vi "Main fref.vi"() -> ()   [LabVIEW 2014]
uses:
  <vilib>/Utility/config.llb/NI_LVConfig.lvlib
  <vilib>/Utility/config.llb/Write Key (String).vi
  <vilib>/Utility/miscctls.llb/LVBoundsTypeDef.ctl
  <vilib>/Utility/miscctls.llb/LVRowAndColumnTypeDef.ctl
  <vilib>/Utility/config.llb/Read Key (String).vi
  TcpConnect/Ctrl/Type.ctl
  user32.dll
  <vilib>/Instr/_visa.llb/VISA Configure Serial Port (Instr).vi
  <vilib>/vision/Image Controls.llb/IMAQ Image.ctl
panel:
  out "螺栓6读取错误":bool
  in  "螺栓6扭矩读取":bool
  in  "扫码保存图片过程":u8
  out "error out 9":errorcluster
  out "error out 8":errorcluster
  out "扭矩/角度":string[][](array[string])
  out "error out 7":errorcluster
  out "error out 5":errorcluster
  out "error out 6":errorcluster
  out "error out 3":errorcluster
  in  "启动python":dbl
  out "产品型号选择":i16
  out "螺栓数量":i16
  out "螺栓5读取错误":bool
  out "螺栓4读取错误":bool
  out "螺栓3读取错误":bool
  out "螺栓2读取错误":bool
  out "螺栓1读取错误":bool
  out "螺栓0读取错误":bool
  in  "螺栓0扭矩读取":bool
  in  "螺栓1扭矩读取":bool
  in  "螺栓2扭矩读取":bool
  in  "螺栓3扭矩读取":bool
  in  "螺栓4扭矩读取":bool
  in  "螺栓5扭矩读取":bool
  in  "复位":bool
  in  "拍照复位信号":bool
  in  "扫码复位信号":bool
  in  "扭矩保存过程":u8
  out "角度字符串":string
  out "扭矩字符串":string
  out "读到的数据":string
  in  "错误输入（无错误） 2":errorcluster caption="错误输入（无错误）"
  out "错误输出 2":errorcluster caption="错误输出"
  in  "拍照存储过程":u8
  in  "开始拍照":bool
  out "图片保存路径":string
  out "error out 4":errorcluster
  in  "Image":T1
  out "扫码NG":bool
  out "扫码OK":bool
  in  "扫码复位":bool
  in  "开始扫码":bool
  out "错误输出":errorcluster
  in  "错误输入（无错误）":errorcluster
  out "当日序号":string
  in  "记录流程":i8
  out "error out":errorcluster caption="错误输出"
  in  "活动单元格:活动单元格 5":T2 caption="活动单元格:活动单元格"
  in  "活动单元格:活动单元格 4":T2 caption="活动单元格:活动单元格"
  in  "活动单元格:活动单元格 3":T2 caption="活动单元格:活动单元格"
  in  "修改确认流程":dbl
  in  "登录过程":dbl
  in  "活动单元格:活动单元格":T2
  in  "选项卡控件":enum32{"操作页面", "设置页面"}(tab)
  out "扭矩7合格":bool
  out "正在拧紧图像（二维码绑定）":T1(plugin-control) caption="正在"
  in  "扭矩角度表格":string[][](table)
  out "拍照合格":bool
  out "扭矩5合格":bool
  out "扭矩6合格":bool
  out "今日合格":string
  out "今日总数":string
  in  "已选产品":string[][](table)
  in  "作业员 Operator":u16(ring) items=["张三", "", "", "", "", "", "", "", "", ""]
  out "二维码":string
  in  "表格":string[][](table)
  out "扭矩4合格":bool
  out "扭矩2合格":bool
  out "扭矩1合格":bool
  out "扭矩3合格":bool
  out "待拧紧前识别图像":T1(plugin-control)
  out "实时图像":T1(plugin-control)
  out "二维码长度":i32
  out "二维码对应程序号":i16
  in  "用户登录":bool
  in  "密码":string
  in  "用户名":string
  in  "用户退出":bool
  in  "产品参数列表（点击表格内任意位置，即可选中所对应产品）":string[][](table)
  in  "程序选择确定":bool
  in  "作业员列表":string[][](table)
  out "字符串":string
types:
  T1 = typedef "IMAQ Image.ctl" = refnum<image>
  T2 = typedef "LVRowAndColumnTypeDef.ctl" = cluster{"Row":i32, "Column":i32}
  T3 = typedef "Type.ctl" = enum16{"Init", "Loop", "Write", "Read", "Exit", "Open", "Close"}
  T4 = typedef "NI_LVConfig.lvlib/Config Data RefNum.ctl" = refnum<k1>
  T5 = cluster{"Name":string, "Type":enum16{"Line", "Broken Line", "Free Hand Line", "Rotated Rectangle", "Oval", "Polygon", "Free Hand", "Bitmap", "Text"}, "Coordinates":i32[], "Colors":u32[], "Drawing Mode":u32, "Text":string, "Results":cluster{"Process ID":string, "Measure":u16, "Name":string, "String Format":u16, "Width":i16, "Precision":i16, "True String":string, "False String":string}[], "Font, Size & Style":cluster{"Desired Font (Application)":enum16{"User-specified Font", "Application Font", "System Font", "Dialog Font"}, "[User-specified Font]":cluster{"Font Name":string, "Size":i16, "Strikeout?":bool, "Italic?":bool, "Underline?":bool, "Outline?":bool, "Shadow?":bool, "Bold?":bool, "Rotation Angle":dbl}, "Horizontal Alignment":i16, "Vertical Alignment":i16}, "Image File Path":path, "Use Keying Color":bool}[]
  T6 = cluster{"Global Rectangle":i32[], "Contours":cluster{"ID":enum32{"External", "Internal"}, "Type":u32, "Coordinates":i32[]}[]}
  T7 = cluster{"Name":string, "Type":enum16{"Line", "Broken Line", "Free Hand Line", "Rotated Rectangle", "Oval", "Polygon", "Free Hand", "Bitmap", "Text"}, "Coordinates":i32[], "Colors":u32[], "Drawing Mode":u32, "Text":string, "Results":cluster{"Process ID":string, "Measure":u16, "Name":string, "String Format":u16, "Width":i16, "Precision":i16, "True String":string, "False String":string}[], "Font, Size & Style":cluster{"Desired Font (Application)":enum16{"User-specified Font", "Application Font", "System Font", "Dialog Font"}, "[User-specified Font]":cluster{"Font Name":string, "Size":i16, "Strikeout?":bool, "Italic?":bool, "Underline?":bool, "Outline?":bool, "Shadow?":bool, "Bold?":bool, "Rotation Angle":dbl}, "Horizontal Alignment":i16, "Vertical Alignment":i16}, "Image File Path":path, "Use Keying Color":bool}
  T8 = enum16{"Line", "Broken Line", "Free Hand Line", "Rotated Rectangle", "Oval", "Polygon", "Free Hand", "Bitmap", "Text"}
  T9 = cluster{"Process ID":string, "Measure":u16, "Name":string, "String Format":u16, "Width":i16, "Precision":i16, "True String":string, "False String":string}[]
  T10 = cluster{"Desired Font (Application)":enum16{"User-specified Font", "Application Font", "System Font", "Dialog Font"}, "[User-specified Font]":cluster{"Font Name":string, "Size":i16, "Strikeout?":bool, "Italic?":bool, "Underline?":bool, "Outline?":bool, "Shadow?":bool, "Bold?":bool, "Rotation Angle":dbl}, "Horizontal Alignment":i16, "Vertical Alignment":i16}
  T11 = enum16{"Standard", "Buffered", "CRLF", "Immediate"}
  T12 = typedef "LVBoundsTypeDef.ctl" = cluster{"Width":u32, "Height":u32}
  T13 = typedef "LVPoint32TypeDef.ctl" = cluster{"Horizontal":i32, "Vertical":i32}
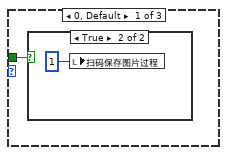
[diagram p2: hidden frame]
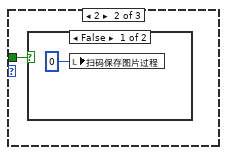
[diagram p4: hidden frame]
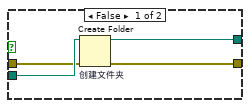
[diagram p6: hidden frame]
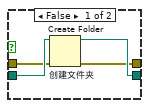
[diagram p7: hidden frame]
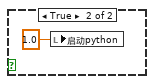
[diagram p8: hidden frame]
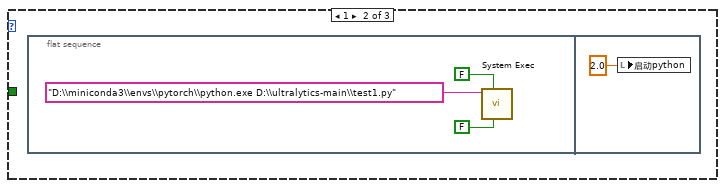
[diagram p9: hidden frame]
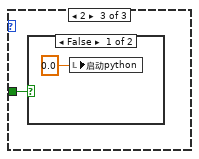
[diagram p10: hidden frame]
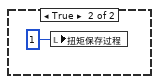
[diagram p14: hidden frame]
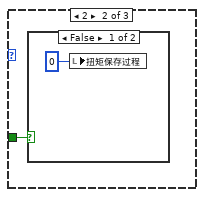
[diagram p15: hidden frame]
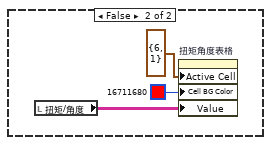
[diagram p18: hidden frame]
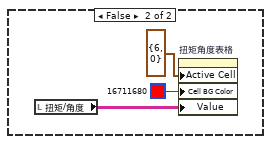
[diagram p19: hidden frame]
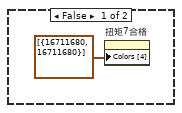
[diagram p20: hidden frame]
diagram:
  n1 = flat-sequence {
    frame #0 {
      w16 = 0
      w14 = 0 items=["NULL"]
      n2 = call "IMAQ Create"("Image Name"="untitled") -> ("New Image"=w25:T1, "error out"=w21:errorcluster)  [unwired: 4 in]
      n3 = call "IMAQ ReadFile 2"("File Path"=path "d:/aotecar.jpg", "error in (no error)"=w21, "Image"=w25) -> ("error out"=w22:errorcluster, "Image Out"=w24:T1)  [unwired: 4 in, 3 out]
      n4 = dll-call lib="user32.dll" fn="FindWindowA" label="FindWindow"("lpszClassName"=w14, "lpszWindowName"="Main.vi") -> ("hWnd"=w18:u32)  [unwired: 5 in, 2 out]
      n5 = call-poly "IMAQ Write File 2"("error in (no error)"=w22, "File Path"=path "d:/image.jpg", "Image"=w24) -> ("Image Out (duplicate)"=w19:T1)  [unwired: 7 in, 1 out]
      n6 = call <vilib>:"System Exec.vi"("run minimized? (F)"=TRUE, "wait until completion? (T)"=FALSE, "command line"="taskkill /F /IM python.exe") -> ()  [unwired: 5 in, 4 out]
      n7 = dll-call lib="USER32.DLL" fn="SetWindowPos"("hWnd"=w18, "hWndInsertAfter"=-1, "left"=w16, "top"=w16, "width"=w16, "height"=w16, "fuFlags"=u32 3) -> ()  [unwired: 11 in, 2 out]
      n8 = local write "待拧紧前识别图像"(w19) -> ()
    }
    frame #1 {
      n9 = Wait (ms)(milliseconds to wait=u32 2000 ("等待时间（毫秒）")) -> ()  [unwired: 1 out]
    }
    frame #2 {
      n10 = while {
        stop <- FALSE stop-if-true
        n11 = call "Get Task List 2.vi"() -> ("names of application windows"=w37:string[])  [unwired: 6 in, 1 out]
        n12 = for {
          N: 10 -> [_]
          tunnel: w37 -> [w47]
          shift-right: [w41] -> w35
          shift-left: 0 -> [w42]
          i -> [w40]
          n13 = Index Array(array=w47, index=w40) -> (element=w46:string)
          n14 = Search and Replace String(case sensitive?=TRUE ("忽略大小写？(F)"), input string=w46, search string="python" ("搜索字符串")) -> (number of replacements=w43:i32)  [unwired: 5 in, 3 out]
          n15 = Add(x=w42, y=w43) -> (x+y=w41:i32)
        }
        n16 = Wait (ms)(milliseconds to wait=u32 1000 ("等待时间（毫秒）")) -> ()  [unwired: 1 out]
        n17 = Equal?(x=w35, y=0) -> (x = y?=w33:bool)
        n18 = case shown="0, 默认" "启动python" {
          tunnel: w33 -> [w48 _ w54]
          frame 0, Default {
            n19 = case shown="False" w48 {
              frame False {
              }
              frame True {
                n20 = local write "启动python"(1.0 ("启动python")) -> ()
              }
            }
          }
          frame 1 {
            n21 = flat-sequence {
              frame #0 {
                n22 = call <vilib>:"System Exec.vi"("run minimized? (F)"=FALSE, "wait until completion? (T)"=FALSE, "command line"="D:\\miniconda3\\envs\\pytorch\\python.exe D:\\ultralytics-main\\test1.py") -> ()  [unwired: 5 in, 4 out]
              }
              frame #1 {
                n23 = local write "启动python"(2.0 ("启动python")) -> ()
              }
            }
          }
          frame 2 {
            n24 = case shown="False" w54 {
              frame False {
                n25 = local write "启动python"(0.0 ("启动python")) -> ()
              }
              frame True {
              }
            }
          }
        }
      }
    }
  }
  n26 = while {
    stop <- FALSE stop-if-true
    n27 = Wait (ms)(milliseconds to wait=u32 100 ("等待时间（毫秒）")) -> ()  [unwired: 1 out]
    n28 = case shown="0, 默认" "修改确认流程" {
      tunnel: "程序选择确定" -> [w60 _ w136]
      frame 0, Default {
        n29 = case shown="False" w60 {
          frame False {
          }
          frame True {
            n30 = local write "修改确认流程"(1.0 ("修改确认流程")) -> ()
          }
        }
      }
      frame 1 {
        n31 = flat-sequence {
          tunnel: [w70] -> w67
          tunnel: [w69] -> w66
          tunnel: w67 -> [w100]
          tunnel: w66 -> [w99]
          tunnel: [w98] -> w65
          tunnel: [w97] -> w64
          tunnel: w65 -> [w132]
          tunnel: w64 -> [w131]
          tunnel: [w131] -> w63
          tunnel: [w132] -> w62
          tunnel: w63 -> [w134]
          tunnel: w62 -> [w133]
          frame #0 {
            n32 = property on="产品参数列表（点击表格内任意位置，即可选中所对应产品）" class="Tbl (严格)"() -> ("Column Headers[]"=w71:string[])  [unwired: 2 in, 2 out]
            n33 = Array Size(array=w71) -> (size(s)=w72:i32)
            n34 = call <vilib>:"Open Config Data.vi"("create file if necessary (T)"=TRUE, "configuration file path"=path "D:/Setup.ini") -> ("error out"=w73:errorcluster, "refnum"=w75:T4)  [unwired: 7 in, 1 out]
            n35 = for {
              N: w72 -> [_]
              tunnel: w75 -> [w82]
              tunnel: w73 -> [w81]
              tunnel: w71 -> [w80]
              tunnel: [w78] -> w70
              tunnel: [w77] -> w69
              i -> [w76]
              n36 = Index Array(array=w80, index=w76) -> (element=w79:string)
              n37 = for {
                N: 100 -> [_]
                tunnel: w82 -> [w96]
                tunnel: [w94] -> w78
                tunnel: w81 -> [w93]
                tunnel: [w92] -> w77
                tunnel: w79 -> [w86]
                tunnel: w76 -> [w85]
                i -> [w91]
                n38 = local read "产品参数列表（点击表格内任意位置，即可选中所对应产品）"() -> (w84:string[][])
                n39 = Increment(x=w91) -> (x+1=w90:i32)
                n40 = Number To Decimal String(number=w90) -> (decimal integer string=w89:string)  [unwired: 1 in]
                n41 = Concatenate Strings(w86, w89) -> (w88:string)
                n42 = Index Array(array=w84, index (row)=w91, index (col)=w85) -> (element=w87:string)
                n43 = call-poly <vilib>:"Write Key.vi"("section"="Setup", "error in (no error)"=w93, "value"=w87, "key"=w88, "refnum"=w96) -> ("error out"=w92:errorcluster, "refnum out"=w94:T4)  [unwired: 4 in, 1 out]
              }
            }
          }
          frame #1 {
            n44 = for {
              N: 35 -> [_]
              tunnel: w100 -> [w130]
              tunnel: [w127] -> w103
              tunnel: w99 -> [w126]
              tunnel: [w125] -> w104
              i -> [w124]
              n45 = Increment(x=w124) -> (x+1=w122:i32)
              n46 = Number To Decimal String(number=w122) -> (decimal integer string=w121:string)  [unwired: 1 in]
              n47 = Concatenate Strings("作业员编码" ("字符串"), w121) -> (w120:string)
              n48 = Index Array(array="作业员列表", index (row)=w124, index (col)=0 ("Column")) -> (element=w118:string)
              n49 = call-poly <vilib>:"Write Key.vi"("section"="Setup", "error in (no error)"=w126, "value"=w118, "key"=w120, "refnum"=w130) -> ("error out"=w125:errorcluster, "refnum out"=w127:T4)  [unwired: 4 in, 1 out]
            }
            n50 = for {
              N: 35 -> [_]
              tunnel: w103 -> [w117]
              tunnel: [w114] -> w98
              tunnel: w104 -> [w113]
              tunnel: [w112] -> w97
              i -> [w111]
              n51 = Increment(x=w111) -> (x+1=w109:i32)
              n52 = local read "作业员列表"() -> (w106:string[][])
              n53 = Number To Decimal String(number=w109) -> (decimal integer string=w108:string)  [unwired: 1 in]
              n54 = Concatenate Strings("作业员姓名" ("字符串"), w108) -> (w107:string)
              n55 = Index Array(array=w106, index (row)=w111, index (col)=1 ("Column")) -> (element=w105:string)
              n56 = call-poly <vilib>:"Write Key.vi"("section"="Setup", "error in (no error)"=w113, "value"=w105, "key"=w107, "refnum"=w117) -> ("error out"=w112:errorcluster, "refnum out"=w114:T4)  [unwired: 4 in, 1 out]
            }
          }
          frame #2 {
          }
          frame #3 {
            n57 = call <vilib>:"Close Config Data.vi"("error in (no error)"=w134, "refnum"=w133) -> ()  [unwired: 8 in, 2 out]
          }
          frame #4 {
            n58 = local write "修改确认流程"(2.0 ("修改确认流程")) -> ()
          }
        }
      }
      frame 2 {
        n59 = case shown="False" w136 {
          frame False {
            n60 = local write "修改确认流程"(0.0 ("修改确认流程")) -> ()
          }
          frame True {
          }
        }
      }
    }
  }
  n61 = disable-structure shown="已启用" {
    frame Disabled {
      n62 = flat-sequence {
        tunnel: [w143] -> w139
        tunnel: [w142] -> w138
        tunnel: w139 -> [w152]
        tunnel: w138 -> [w151]
        frame #0 {
          n63 = call <vilib>:"Open Config Data.vi"("create file if necessary (T)"=TRUE, "configuration file path"=path "D:/Test/Setup.ini") -> ("error out"=w149:errorcluster, "refnum"=w148:T4)  [unwired: 7 in, 1 out]
          n64 = call-poly <vilib>:"Read Key.vi"("section"="Setup", "error in (no error)"=w149, "refnum"=w148) -> ("error out"=w143:errorcluster, "value"=w147:string, "refnum out"=w142:T4, "key"=w140:string)  [unwired: 4 in, 1 out]
          n65 = Write to Text File(file (use dialog)=path "D:/扫码端口号.txt" ("文件（使用对话框）"), text=w147) -> ()  [unwired: 2 in, 3 out]
        }
        frame #1 {
          n66 = call <vilib>:"Close Config Data.vi"("error in (no error)"=w152, "refnum"=w151) -> ("error out"=→"error out":errorcluster)  [unwired: 8 in, 1 out]
        }
        frame #2 {
          n67 = Wait (ms)(milliseconds to wait=u32 2000 ("等待时间（毫秒）")) -> ()  [unwired: 1 out]
        }
        frame #3 {
          n68 = while {
            stop <- w158 stop-if-true
            n69 = Read from Text File(file (use dialog)=path "D:/扫码端口号.txt" ("文件（使用对话框）")) -> (text=w154:string)  [unwired: 3 in, 3 out]
            n70 = VISA Open(VISA resource name=w154) -> (VISA resource name=w156:refnum<visa-resource-name>, error out=w157:errorcluster)  [unwired: 4 in]
            n71 = case shown="错误" w157 {
              tunnel: w156 -> [w187 _]
              tunnel: 9600 -> [w183 _]
              tunnel: [w182 _] -> w162
              tunnel: [w181 _] -> w161
              frame No Error {
                n72 = call-poly "VISA Configure Serial Port"("VISA resource name"=w187, "baud rate (9600)"=w183) -> ("VISA resource name out"=w185:refnum<visa-resource-name>, "error out"=w186:errorcluster)  [unwired: 12 in]
                n73 = VISA Set I/O Buffer Size "VISA设置I/O缓冲区大小"(VISA resource name=w185, size (4096)=u32 20480 ("大小(4096)"), error in (no error)=w186) -> (VISA resource name out=w182:refnum<visa-resource-name>, error out=w181:errorcluster)  [unwired: 1 in]
              }
              frame Error {
                n74 = One Button Dialog(message="ERROR！" ("消息")) -> ()  [unwired: 1 in, 1 out]
              }
            }
            n75 = while {
              tunnel: w162 -> [w166]
              tunnel: w161 -> [w165]
              tunnel: [w172] -> w160
              tunnel: [w171] -> w159
              shift-right: [w170] -> _
              shift-left: _ -> [w169]
              tunnel: [w167] -> w158
              stop <- w167 stop-if-true
              w167 = FALSE
              n76 = Concatenate Strings "连接字符串"(w169) -> (w164:string)  [unwired: 1 in]
              n77 = flat-sequence {
                tunnel: w166 -> [w180]
                tunnel: w165 -> [w179]
                tunnel: [w175] -> w172
                tunnel: [w174] -> w171
                tunnel: [w173] -> w170
                frame #0 {
                  n78 = property class="Instr"(reference=w180, error in=w179) -> (reference out=w178:refnum<visa-resource-name>, error out=w177:errorcluster, "Bytes at Port"=w176:u32)
                  n79 = VISA Read(VISA resource name=w178, byte count=w176, error in (no error)=w177) -> (VISA resource name out=w175:refnum<visa-resource-name>, read buffer=w173:string, error out=w174:errorcluster)  [unwired: 1 out]
                }
              }
              n80 = local write item#-1(w164) -> ()
              n81 = Wait Until Next ms Multiple(millisecond multiple=u32 2 ("毫秒倍数")) -> ()  [unwired: 1 out]
            }
            n82 = VISA Close(VISA resource name=w160, error in (no error)=w159) -> ()  [unwired: 1 out]
          }
        }
      }
    }
    frame Enabled {
    }
  }
  n83 = disable-structure shown="禁用" {
    frame Disabled {
      n84 = while {
        stop <- FALSE stop-if-true
        n85 = local read item#-1() -> (w189)
        n86 = case shown="1" "记录流程" {
          tunnel: w189 -> [w192 _ w288]
          frame 0 {
            n87 = case shown="False" w192 {
              frame False {
              }
              frame True {
                n88 = local write "记录流程"(i8 1 ("耐压测试左")) -> ()
              }
            }
          }
          frame 1 {
            n89 = flat-sequence {
              tunnel: [w198] -> w195
              tunnel: w195 -> [w208]
              tunnel: [w238] -> w194
              tunnel: w194 -> [w273]
              frame #0 {
                n90 = Open/Create/Replace File(file path (use dialog)=path "D:/日期.txt" ("文件（使用对话框）")) -> (refnum out=w205:refnum<file>, error out=w204:errorcluster)  [unwired: 5 in, 1 out]
                n91 = Read from Text File "读取文本文件"(file (use dialog)=w205, error in=w204) -> (refnum out=w197:refnum<file>, text=w201:string, error out=w196:errorcluster)  [unwired: 2 in, 1 out]
                n92 = Close File(refnum=w197, error in=w196) -> ()  [unwired: 2 out]
                n93 = Format Date/Time String(time format string (%c)="%Y%m%d" ("时间格式字符串(%c)")) -> (date/time string=w202:string)  [unwired: 2 in]
                n94 = Decimal String To Number(string=w201) -> (number=w199:i32)  [unwired: 2 in, 1 out]
                n95 = Decimal String To Number(string=w202) -> (number=w200:i32)  [unwired: 2 in, 1 out]
                n96 = Equal?(x=w199, y=w200) -> (x = y?=w198:bool)
              }
              frame #1 {
                n97 = case shown="True" w208 {
                  tunnel: [w209 w221] -> w207
                  frame False {
                    n98 = Number To Decimal String(number=1 ("数字"), width (-)=i16 4 ("宽度(-)")) -> (decimal integer string=w219:string)
                    n99 = call <vilib>:"Space Constant.vi"() -> ("String"=w220:string)
                    n100 = Search and Replace String(replace all?=TRUE ("替换全部？(F)"), input string=w219, search string=w220, replace string="0" ("替换字符串(\"\")")) -> (result string=w209:string)  [unwired: 4 in, 3 out]
                    n101 = Open/Create/Replace File(file path (use dialog)=path "D:/序号.txt" ("文件（使用对话框）")) -> (refnum out=w212:refnum<file>, error out=w211:errorcluster)  [unwired: 5 in, 1 out]
                    n102 = Write to Text File "写入文本文件"(file (use dialog)=w212, text=w209, error in=w211) -> (refnum out=w217:refnum<file>, error out=w218:errorcluster)  [unwired: 1 in, 1 out]
                    n103 = Close File(refnum=w217, error in=w218) -> ()  [unwired: 2 out]
                  }
                  frame True {
                    n104 = Open/Create/Replace File(file path (use dialog)=path "D:/序号.txt" ("文件（使用对话框）")) -> (refnum out=w224:refnum<file>, error out=w225:errorcluster)  [unwired: 5 in, 1 out]
                    n105 = Read from Text File "读取文本文件"(file (use dialog)=w224, error in=w225) -> (refnum out=w222:refnum<file>, text=w229:string, error out=w223:errorcluster)  [unwired: 2 in, 1 out]
                    n106 = Decimal String To Number(string=w229) -> (number=w235:i32)  [unwired: 2 in, 1 out]
                    n107 = Increment(x=w235) -> (x+1=w236:i32)
                    n108 = Number To Decimal String(number=w236, width (-)=i16 4 ("宽度(-)")) -> (decimal integer string=w231:string)
                    n109 = call <vilib>:"Space Constant.vi"() -> ("String"=w234:string)
                    n110 = Search and Replace String(replace all?=TRUE ("替换全部？(F)"), input string=w231, search string=w234, replace string="0" ("替换字符串(\"\")")) -> (result string=w221:string)  [unwired: 4 in, 3 out]
                    n111 = Write to Text File "写入文本文件"(file (use dialog)=w222, text=w221, error in=w223) -> (refnum out=w227:refnum<file>, error out=w228:errorcluster)  [unwired: 1 in, 1 out]
                    n112 = Close File(refnum=w227, error in=w228) -> ()  [unwired: 2 out]
                  }
                }
                "当日序号" <- w207
              }
              frame #2 {
                n113 = Build Path "创建路径"(name or relative path=path "D:/Image" ("基路径")) -> (appended path=w239:path)  [unwired: 1 in]
                n114 = call <vilib>:"Check if File or Folder Exists.vi"("path"=w239) -> ("error out"=w242:errorcluster, "file or folder exists?"=w241:bool, "dup path"=w240:path)  [unwired: 1 in, 7 out]
                n115 = case shown="True" w241 {
                  tunnel: [w243 w246] -> w238
                  tunnel: w240 -> [w245 w246]
                  tunnel: w242 -> [w244 _]
                  frame False {
                    n116 = Create Folder "创建文件夹"(path (use dialog)=w245, error in=w244) -> (created path=w243:path)  [unwired: 3 out]
                  }
                  frame True {
                  }
                }
              }
              frame #3 {
                n117 = Get Date/Time In Seconds "获取日期/时间（秒）"() -> (seconds since 1Jan1904=w271:timestamp)
                n118 = Format Date/Time String(time format string (%c)="%Y%m%d" ("时间格式字符串(%c)")) -> (date/time string=w248:string)  [unwired: 2 in]
                n119 = Open/Create/Replace File(file path (use dialog)=path "D:/日期.txt" ("文件（使用对话框）")) -> (refnum out=w250:refnum<file>, error out=w251:errorcluster)  [unwired: 5 in, 1 out]
                n120 = Path To String(path=w273) -> (string=w281:string)
                n121 = Write to Text File(file (use dialog)=w250, text=w248, error in=w251) -> (refnum out=w253:refnum<file>, error out=w254:errorcluster)  [unwired: 1 in, 1 out]
                n122 = Format Date/Time String(time format string (%c)="%Y-%m-%d" ("时间格式字符串(%c)"), seconds (now)=w271) -> (date/time string=w276:string)  [unwired: 1 in]
                n123 = Close File(refnum=w253, error in=w254) -> ()  [unwired: 2 out]
                n124 = Concatenate Strings(w281, "\\", w276) -> (w275:string)
                n125 = Build Path(name or relative path=w275) -> (appended path=w277:path)  [unwired: 1 in]
                n126 = call <vilib>:"Check if File or Folder Exists.vi"("path"=w277) -> ("error out"=w280:errorcluster, "file or folder exists?"=w279:bool, "dup path"=w278:path)  [unwired: 1 in, 7 out]
                n127 = case shown="False" w279 {
                  tunnel: [w282 w285] -> w264
                  tunnel: w278 -> [w284 w285]
                  tunnel: w280 -> [w283 _]
                  frame False {
                    n128 = Create Folder(path (use dialog)=w284, error in=w283) -> (created path=w282:path)  [unwired: 3 out]
                  }
                  frame True {
                  }
                }
                n129 = Path To String(path=w264) -> (string=w256:string)
                n130 = Format Date/Time String(time format string (%c)="%Y-%m-%d-%H-%M-%S-翅片" ("时间格式字符串(%c)")) -> (date/time string=w262:string)  [unwired: 2 in]
                n131 = Format Date/Time String(time format string (%c)="%Y-%m-%d-%H-%M-%S-O型圈" ("时间格式字符串(%c)")) -> (date/time string=w259:string)  [unwired: 2 in]
                n132 = Concatenate Strings(w256, "\\", w262) -> (w265:string)
                n133 = Concatenate Strings(w256, "\\", w259) -> (w260:string)
                n134 = Build Path(name or relative path=w265) -> (appended path=w261:path)  [unwired: 1 in]
                n135 = Build Path(name or relative path=w260) -> (appended path=w255:path)  [unwired: 1 in]
                n136 = call-poly "IMAQ Write File 2"("File Path"=w261, "Image"="Image") -> ("error out"=w269:errorcluster, "Image Out (duplicate)"=w270:T1)  [unwired: 8 in]
                n137 = call-poly "IMAQ Write File 2"("File Path"=w255, "Image"="Image") -> ("error out"=w268:errorcluster, "Image Out (duplicate)"=w267:T1)  [unwired: 8 in]
                n138 = call "IMAQ Dispose"("Image"=w270, "error in (no error)"=w269) -> ()  [unwired: 4 in, 1 out]
                n139 = call "IMAQ Dispose"("Image"=w267, "error in (no error)"=w268) -> ()  [unwired: 4 in, 1 out]
              }
              frame #4 {
                n140 = Wait (ms)(milliseconds to wait=u32 1000 ("等待时间（毫秒）")) -> ()  [unwired: 1 out]
              }
              frame #5 {
              }
              frame #6 {
                n141 = local write "记录流程"(i8 2 ("耐压测试左")) -> ()
              }
            }
          }
          frame 2, Default {
            n142 = case shown="True" w288 {
              frame False {
                n143 = local write "记录流程"(i8 0 ("耐压测试左")) -> ()
              }
              frame True {
              }
            }
          }
        }
      }
    }
    frame Enabled {
    }
  }
  n144 = while {
    tunnel: [w296] -> w5
    tunnel: [w295] -> w4
    stop <- w299 stop-if-true
    w303 = u32 0 items=["Grayscale", "Binary", "Gradient", "Rainbow", "Temperature", "User Defined", "Binary 16 Bit", "Gradient 16 Bit", "Rainbow 16 Bit", "Temperature 16 Bit", "User Defined 16 Bit"] ("Palette Type")
    w304 = T6 {"Global Rectangle"=[545, -12, 2261, 2048], "Contours"=[{"ID"=enum."External", "Type"=3, "Coordinates"=[545, -12, 2261, 2048]}]}  # ROI Descriptor
    n145 = Wait (ms)(milliseconds to wait=u32 150 ("等待时间（毫秒）")) -> ()  [unwired: 1 out]
    n146 = Index Array(array=T5 [{"Name"="Text 1", "Type"=enum."Text", "Coordinates"=[900, 1900], "Colors"=[16711680, 16777216], "Drawing Mode"=0, "Text"="%Y%m%d_%H_%M_%Sour Text", "Results"=[], "Font, Size & Style"={"Desired Font (Application)"=enum."User-specified Font", "[User-specified Font]"={"Font Name"="Tahoma", "Size"=100, "Strikeout?"=FALSE, "Italic?"=FALSE, "Underline?"=FALSE, "Outline?"=FALSE, "Shadow?"=FALSE, "Bold?"=FALSE, "Rotation Angle"=0.0}, "Horizontal Alignment"=0, "Vertical Alignment"=0}, "Image File Path"=path "", "Use Keying Color"=FALSE}] ("Parameters"), index=0 ("索引")) -> (element=w311:T7)
    n147 = Unbundle By Name(w311) -> ("Name"=w312:string, "Type"=w313:T8, "Coordinates"=w314:i32[], "Colors"=w315:u32[], "Drawing Mode"=w316:u32, "Results"=w319:T9, "Font, Size & Style"=w320:T10, "Image File Path"=w321:path, "Use Keying Color"=w322:bool)  [unwired: 1 out]
    n148 = Format Date/Time String(time format string (%c)="%Y%m%d_%H_%M_%S" ("时间格式字符串(%c)")) -> (date/time string=w317:string)  [unwired: 2 in]
    n149 = Bundle By Name(cluster=w311, "Name"=w312, "Type"=w313, "Coordinates"=w314, "Colors"=w315, "Drawing Mode"=w316, "Text"=w317, "Results"=w319, "Font, Size & Style"=w320, "Image File Path"=w321, "Use Keying Color"=w322) -> (w323:T7)
    n150 = call "Vision Acquisition"() -> ("Image Out"=w301:T1, "Stopped"=w299:bool, "error out"=w300:errorcluster)  [unwired: 25 in]
    n151 = Build Array(w323) -> (w324:T5)
    n152 = call <vilib>:"IVA Mask from ROI.vi"("Shrink"=TRUE, "ROI Descriptor"=w304, "error in (no error)"=w300, "Out / In"=FALSE, "Image Src"=w301) -> ("error out"=w308:errorcluster, "Image Out"=w307:T1)  [unwired: 5 out]
    n153 = call <vilib>:"IVA Overlay - Overlay.vi"("error in (no error)"=w308, "Parameters"=w324, "Image In"=w307) -> ("error out"=w291:errorcluster, "Image Out"=w293:T1)  [unwired: 7 out]
    n154 = call "IMAQ Merge Overlay"("error in (no error)"=w291, "Image Src"=w293) -> ("error out"=w290:errorcluster, "Image Dst Out"=w292:T1)  [unwired: 8 in]
    "实时图像" <- w292
    n155 = property on="实时图像" class="ImageControl"(error in=w290, "Palette:Palette Type"=w303) -> (error out=→"error out 7":errorcluster)  [unwired: 1 in, 1 out]
    n156 = call-poly "IMAQ Write File 2"("Image Quality"=u32 250, "File Path"=path "d:/source.jpg", "Image"=w292) -> ("error out"=w296:errorcluster, "Image Out (duplicate)"=w295:T1)  [unwired: 7 in]
  }
  n157 = while {
    tunnel: [w326] -> w2
    tunnel: [w325] -> w1
    stop <- FALSE stop-if-true
    n158 = Wait (ms)(milliseconds to wait=u32 100 ("等待时间（毫秒）")) -> ()  [unwired: 1 out]
    n159 = local read "扫码OK"() -> (w327:bool)
    n160 = case shown="1" "扫码保存图片过程" {
      tunnel: w327 -> [w331 w333 _]
      tunnel: [_ _ w336] -> w326
      tunnel: [_ _ w335] -> w325
      frame 0, Default {
        n161 = case shown="True" w331 {
          frame False {
          }
          frame True {
            n162 = local write "扫码保存图片过程"(u8 1 ("扫码保存图片过程")) -> ()
          }
        }
      }
      frame 2 {
        n163 = case shown="False" w333 {
          frame False {
            n164 = local write "扫码保存图片过程"(u8 0 ("扫码保存图片过程")) -> ()
          }
          frame True {
          }
        }
      }
      frame 1 {
        n165 = flat-sequence {
          tunnel: [w361] -> w336
          tunnel: [w360] -> w335
          frame #0 {
            w338 = FALSE
            n166 = Initialize Array("", 7 ("维数大小"), 2 ("维数大小")) -> (w349:string[][])
            n167 = for {
              N: 7 -> [_]
              i -> [w350]
              n168 = for {
                N: 2 -> [_]
                tunnel: w350 -> [w357]
                i -> [w358]
                n169 = Bundle(w357, w358) -> (w356:cluster{i32, i32})  [unwired: 1 in]
                n170 = Initialize Array("", 7 ("维数大小"), 2 ("维数大小")) -> (w354:string[][])
                n171 = property on="扭矩角度表格" class="Tbl (严格)"("Active Cell"=w356, "Cell BG Color"=u32 16448250 ("活动单元格:单元格背景色"), "Value"=w354) -> ()  [unwired: 2 in, 2 out]
              }
            }
            n172 = local write "扭矩1合格"(w338) -> ()
            n173 = local write "扭矩2合格"(w338) -> ()
            n174 = local write "扭矩3合格"(w338) -> ()
            n175 = local write "扭矩4合格"(w338) -> ()
            n176 = local write "扭矩5合格"(w338) -> ()
            n177 = local write "扭矩6合格"(w338) -> ()
            n178 = property on="扭矩6合格" class="Bool (严格)"("Colors [4]"=cluster{u32, u32}[] [{12369084, 12369084}] ("颜色[4]")) -> ()  [unwired: 2 in, 2 out]
            n179 = local write "扭矩/角度"(w349) -> ()
            n180 = property on="扭矩4合格" class="Bool (严格)"("Colors [4]"=cluster{u32, u32}[] [{12369084, 12369084}] ("颜色[4]")) -> ()  [unwired: 2 in, 2 out]
            n181 = property on="扭矩5合格" class="Bool (严格)"("Colors [4]"=cluster{u32, u32}[] [{12369084, 12369084}] ("颜色[4]")) -> ()  [unwired: 2 in, 2 out]
            n182 = property on="扭矩3合格" class="Bool (严格)"("Colors [4]"=cluster{u32, u32}[] [{12369084, 12369084}] ("颜色[4]")) -> ()  [unwired: 2 in, 2 out]
            n183 = property on="扭矩2合格" class="Bool (严格)"("Colors [4]"=cluster{u32, u32}[] [{12369084, 12369084}] ("颜色[4]")) -> ()  [unwired: 2 in, 2 out]
            n184 = property on="扭矩1合格" class="Bool (严格)"("Colors [4]"=cluster{u32, u32}[] [{12369084, 12369084}] ("颜色[4]")) -> ()  [unwired: 2 in, 2 out]
            n185 = local write "扭矩7合格"(w338) -> ()
            n186 = property on="扭矩7合格" class="Bool (严格)"("Colors [4]"=cluster{u32, u32}[] [{12369084, 12369084}] ("颜色[4]")) -> ()  [unwired: 2 in, 2 out]
          }
          frame #1 {
            n187 = String To Path(string="D:\\Image\\" ("字符串")) -> (path=w400:path)
            n188 = Format Date/Time String(time format string (%c)="%Y%m") -> (date/time string=w399:string)  [unwired: 2 in]
            n189 = Build Path(base path=w400, name or relative path=w399) -> (appended path=w398:path)
            n190 = call <vilib>:"Check if File or Folder Exists.vi"("path"=w398) -> ("error out"=w405:errorcluster, "file or folder exists?"=w397:bool)  [unwired: 8 in, 1 out]
            n191 = case shown="True" w397 {
              tunnel: w398 -> [w420 w422]
              tunnel: [w419 w422] -> w403
              tunnel: w405 -> [w418 w421]
              tunnel: [w417 w421] -> w406
              frame False {
                n192 = Create Folder "创建文件夹"(path (use dialog)=w420, error in=w418) -> (created path=w419:path, error out=w417:errorcluster)  [unwired: 1 in, 1 out]
              }
              frame True {
              }
            }
            n193 = Format Date/Time String(time format string (%c)="%d") -> (date/time string=w402:string)  [unwired: 2 in]
            n194 = Build Path(base path=w403, name or relative path=w402) -> (appended path=w404:path)
            n195 = Index Array(array=T5 [{"Name"="Text 1", "Type"=enum."Text", "Coordinates"=[100, 2000], "Colors"=[16711680, 16777216], "Drawing Mode"=0, "Text"="%Y%m%d_%H_%M_%Sour Text", "Results"=[], "Font, Size & Style"={"Desired Font (Application)"=enum."User-specified Font", "[User-specified Font]"={"Font Name"="Tahoma", "Size"=100, "Strikeout?"=FALSE, "Italic?"=FALSE, "Underline?"=FALSE, "Outline?"=FALSE, "Shadow?"=FALSE, "Bold?"=FALSE, "Rotation Angle"=0.0}, "Horizontal Alignment"=0, "Vertical Alignment"=0}, "Image File Path"=path "", "Use Keying Color"=FALSE}] ("Parameters"), index=0 ("索引")) -> (element=w374:T7)
            n196 = Unbundle By Name(w374) -> ("Name"=w375:string, "Type"=w376:T8, "Coordinates"=w377:i32[], "Colors"=w378:u32[], "Drawing Mode"=w379:u32, "Results"=w380:T9, "Font, Size & Style"=w381:T10, "Image File Path"=w382:path, "Use Keying Color"=w383:bool)  [unwired: 1 out]
            n197 = call <vilib>:"Check if File or Folder Exists.vi"("error in (no error)"=w406, "path"=w404) -> ("error out"=w407:errorcluster, "file or folder exists?"=w401:bool)  [unwired: 7 in, 1 out]
            n198 = local read "二维码长度"() -> (w364:i32)
            n199 = case shown="True" w401 {
              tunnel: w404 -> [w414 w415]
              tunnel: [w413 w415] -> w395
              tunnel: w407 -> [w412 w416]
              tunnel: [w411 w416] -> _
              frame False {
                n200 = Create Folder "创建文件夹"(path (use dialog)=w414, error in=w412) -> (created path=w413:path, error out=w411:errorcluster)  [unwired: 1 in, 1 out]
              }
              frame True {
              }
            }
            n201 = local read "二维码"() -> (w365:string)
            n202 = local read "二维码"() -> (w369:string)
            n203 = Bundle By Name(cluster=w374, "Name"=w375, "Type"=w376, "Coordinates"=w377, "Colors"=w378, "Drawing Mode"=w379, "Text"=w369, "Results"=w380, "Font, Size & Style"=w381, "Image File Path"=w382, "Use Keying Color"=w383) -> (w384:T7)
            n204 = String Subset(string=w365, length (rest)=w364) -> (substring=w366:string)  [unwired: 1 in]
            n205 = Format Date/Time String(time format string (%c)="%Y%m%d_%H_%M_%S") -> (date/time string=w394:string)  [unwired: 2 in]
            n206 = call "IMAQ Create"("Image Name"="untitled3") -> ("New Image"=w409:T1, "error out"=w410:errorcluster)  [unwired: 4 in]
            n207 = Build Array(w384) -> (w385:T5)
            n208 = call "IMAQ ReadFile 2"("File Path"=path "d:/buffer.jpg", "error in (no error)"=w410, "Image"=w409) -> ("error out"=w362:errorcluster, "Image Out"=w363:T1)  [unwired: 4 in, 3 out]
            n209 = call <vilib>:"IVA Overlay - Overlay.vi"("error in (no error)"=w362, "Parameters"=w385, "Image In"=w363) -> ("error out"=w372:errorcluster, "Image Out"=w373:T1)  [unwired: 7 out]
            n210 = Concatenate Strings(w366, w394, ".JPEG" ("字符串")) -> (w408:string)
            n211 = Build Path(base path=w395, name or relative path=w408) -> (appended path=w393:path)
            n212 = call "IMAQ Merge Overlay"("error in (no error)"=w372, "Image Src"=w373) -> ("error out"=w367:errorcluster, "Image Dst Out"=w368:T1)  [unwired: 8 in]
            n213 = Path To String(path=w393) -> (string=→"图片保存路径":string)
            n214 = call-poly "IMAQ Write File 2"("error in (no error)"=w367, "File Path"=w393, "Image"=w368) -> ("error out"=w360:errorcluster, "Image Out (duplicate)"=w361:T1)  [unwired: 7 in]
            "正在拧紧图像（二维码绑定）" <- w361
          }
          frame #2 {
            n215 = local write "扫码保存图片过程"(u8 2 ("扫码保存图片过程")) -> ()
          }
        }
      }
    }
  }
  n216 = while {
    stop <- FALSE stop-if-true
    n217 = Wait (ms)(milliseconds to wait=u32 50 ("等待时间（毫秒）")) -> ()  [unwired: 1 out]
    n218 = case shown="1" "拍照存储过程" {
      tunnel: "开始拍照" -> [w428 w430 _]
      frame 0, Default {
        n219 = case shown="True" w428 {
          frame False {
          }
          frame True {
            n220 = local write "拍照存储过程"(u8 1 ("拍照存储过程")) -> ()
          }
        }
      }
      frame 2 {
        n221 = case shown="False" w430 {
          frame False {
            n222 = local write "拍照存储过程"(u8 0 ("拍照存储过程")) -> ()
          }
          frame True {
          }
        }
      }
      frame 1 {
        n223 = flat-sequence {
          frame #0 {
            n224 = Wait (ms)(milliseconds to wait=u32 3000 ("等待时间（毫秒）")) -> ()  [unwired: 1 out]
          }
          frame #1 {
            n225 = call "IMAQ Create"("Image Name"="untitled2") -> ("New Image"=w435:T1, "error out"=w436:errorcluster)  [unwired: 4 in]
            n226 = call "IMAQ ReadFile 2"("File Path"=path "d:/image.jpg", "error in (no error)"=w436, "Image"=w435) -> ("error out"=→"error out 3":errorcluster, "Image Out"=→"待拧紧前识别图像":T1)  [unwired: 4 in, 3 out]
          }
          frame #2 {
            n227 = for {
              N: 3 -> [_]
              tunnel: [w499] -> w483
              n228 = local read "已选产品"() -> (w502:string[][])
              n229 = Read from Text File(file (use dialog)=path "d:/image.txt" ("文件（使用对话框）")) -> (text=w506:string, error out=w505:errorcluster)  [unwired: 3 in, 2 out]
              n230 = Index Array(array=w502, index (row)=0 ("禁用的索引 (行)"), index (col)=7 ("禁用的索引 (列)")) -> (element=w503:string)
              n231 = Decimal String To Number(string=w503) -> (number=w497:i32)  [unwired: 2 in, 1 out]
              n232 = Search and Replace String(replace all?=TRUE ("替换全部？(F)"), input string=w506, search string="screw" ("Image Name"), error in=w505) -> (number of replacements=w498:i32)  [unwired: 4 in, 3 out]
              n233 = Equal?(x=w498, y=w497) -> (x = y?=w499:bool)
            }
            n234 = call "IMAQ Create"("Image Name"="untitled5") -> ("New Image"=w472:T1, "error out"=w479:errorcluster)  [unwired: 4 in]
            n235 = String To Path(string="D:\\Image\\temp\\" ("字符串")) -> (path=w465:path)
            n236 = call "IMAQ ReadFile 2"("File Path"=path "d:/source.jpg", "error in (no error)"=w479, "Image"=w472) -> ("error out"=w477:errorcluster, "Image Out"=w478:T1)  [unwired: 4 in, 3 out]
            n237 = Format Date/Time String(time format string (%c)="%Y%m") -> (date/time string=w466:string)  [unwired: 2 in]
            n238 = Build Path(base path=w465, name or relative path=w466) -> (appended path=w467:path)
            n239 = call-poly "IMAQ Write File 2"("error in (no error)"=w477, "File Path"=path "d:/buffer.jpg", "Image"=w478) -> ("error out"=w481:errorcluster, "Image Out (duplicate)"=w474:T1)  [unwired: 7 in]
            n240 = call <vilib>:"Check if File or Folder Exists.vi"("path"=w467) -> ("error out"=w460:errorcluster, "file or folder exists?"=w468:bool)  [unwired: 8 in, 1 out]
            n241 = case shown="True" w468 {
              tunnel: w467 -> [w493 w495]
              tunnel: [w492 w495] -> w462
              tunnel: w460 -> [w491 w494]
              tunnel: [w490 w494] -> w459
              frame False {
                n242 = Create Folder "创建文件夹"(path (use dialog)=w493, error in=w491) -> (created path=w492:path, error out=w490:errorcluster)  [unwired: 1 in, 1 out]
              }
              frame True {
              }
            }
            n243 = call "IMAQ Dispose"("Image"=w474, "error in (no error)"=w481) -> ("error out"=→"error out 8":errorcluster)  [unwired: 4 in]
            n244 = case shown="False" w483 {
              frame True {
                n245 = shared-variable "我的电脑\\opc.lvlib\\相机识别NG"(FALSE ("相机识别OK")) -> ()  [unwired: 1 in, 1 out]
                n246 = shared-variable "我的电脑\\opc.lvlib\\相机识别OK"(TRUE ("相机识别OK")) -> ()  [unwired: 1 in, 1 out]
                n247 = property on="拍照合格" class="Bool (严格)"("Colors [4]"=cluster{u32, u32}[] [{6618880, 6618880}] ("颜色[4]")) -> ()  [unwired: 2 in, 2 out]
              }
              frame False {
                n248 = shared-variable "我的电脑\\opc.lvlib\\相机识别OK"(FALSE ("相机识别OK")) -> ()  [unwired: 1 in, 1 out]
                n249 = shared-variable "我的电脑\\opc.lvlib\\相机识别NG"(TRUE ("相机识别OK")) -> ()  [unwired: 1 in, 1 out]
                n250 = property on="拍照合格" class="Bool (严格)"("Colors [4]"=cluster{u32, u32}[] [{16711680, 16711680}] ("颜色[4]")) -> ()  [unwired: 2 in, 2 out]
                n251 = String To Path(string="D:\\Image\\NG\\" ("字符串")) -> (path=w517:path)
                n252 = Format Date/Time String(time format string (%c)="%Y%m") -> (date/time string=w516:string)  [unwired: 2 in]
                n253 = Build Path(base path=w517, name or relative path=w516) -> (appended path=w515:path)
                n254 = call <vilib>:"Check if File or Folder Exists.vi"("path"=w515) -> ("error out"=w522:errorcluster, "file or folder exists?"=w514:bool)  [unwired: 8 in, 1 out]
                n255 = case shown="True" w514 {
                  tunnel: w515 -> [w556 w558]
                  tunnel: [w555 w558] -> w520
                  tunnel: w522 -> [w554 w557]
                  tunnel: [w553 w557] -> w523
                  frame False {
                    n256 = Create Folder "创建文件夹"(path (use dialog)=w556, error in=w554) -> (created path=w555:path, error out=w553:errorcluster)  [unwired: 1 in, 1 out]
                  }
                  frame True {
                  }
                }
                n257 = Format Date/Time String(time format string (%c)="%d") -> (date/time string=w519:string)  [unwired: 2 in]
                n258 = Build Path(base path=w520, name or relative path=w519) -> (appended path=w521:path)
                n259 = call <vilib>:"Check if File or Folder Exists.vi"("error in (no error)"=w523, "path"=w521) -> ("error out"=w524:errorcluster, "file or folder exists?"=w518:bool)  [unwired: 7 in, 1 out]
                n260 = local read "已选产品"() -> (w531:string[][])
                n261 = case shown="True" w518 {
                  tunnel: w521 -> [w550 w551]
                  tunnel: [w549 w551] -> w513
                  tunnel: w524 -> [w548 w552]
                  tunnel: [w547 w552] -> _
                  frame False {
                    n262 = Create Folder "创建文件夹"(path (use dialog)=w550, error in=w548) -> (created path=w549:path, error out=w547:errorcluster)  [unwired: 1 in, 1 out]
                  }
                  frame True {
                  }
                }
                n263 = Format Date/Time String(time format string (%c)="%Y%m%d_%H_%M_%S") -> (date/time string=w512:string)  [unwired: 2 in]
                n264 = Index Array(array=w531, index (row)=0 ("禁用的索引 (行)"), index (col)=0 ("禁用的索引 (列)")) -> (element=w534:string)
                n265 = Concatenate Strings(w534, w512, ".JPEG" ("字符串")) -> (w525:string)
                n266 = call "IMAQ Create"("Image Name"="untitled4") -> ("New Image"=w539:T1, "error out"=w540:errorcluster)  [unwired: 4 in]
                n267 = Build Path(base path=w513, name or relative path=w525) -> (appended path=w511:path)
                n268 = call "IMAQ ReadFile 2"("File Path"=path "d:/image.jpg", "error in (no error)"=w540, "Image"=w539) -> ("error out"=w542:errorcluster, "Image Out"=w541:T1)  [unwired: 4 in, 3 out]
                n269 = call-poly "IMAQ Write File 2"("error in (no error)"=w542, "File Path"=w511, "Image"=w541) -> ("error out"=w536:errorcluster, "Image Out (duplicate)"=w535:T1)  [unwired: 7 in]
                n270 = call "IMAQ Dispose"("Image"=w535, "error in (no error)"=w536) -> ("error out"=→"error out 5":errorcluster)  [unwired: 4 in]
              }
            }
            n271 = Format Date/Time String(time format string (%c)="%d") -> (date/time string=w463:string)  [unwired: 2 in]
            n272 = Build Path(base path=w462, name or relative path=w463) -> (appended path=w461:path)
            n273 = call <vilib>:"Check if File or Folder Exists.vi"("error in (no error)"=w459, "path"=w461) -> ("error out"=w458:errorcluster, "file or folder exists?"=w464:bool)  [unwired: 7 in, 1 out]
            n274 = local read "已选产品"() -> (w451:string[][])
            n275 = case shown="True" w464 {
              tunnel: w461 -> [w487 w488]
              tunnel: [w486 w488] -> w469
              tunnel: w458 -> [w485 w489]
              tunnel: [w484 w489] -> _
              frame False {
                n276 = Create Folder "创建文件夹"(path (use dialog)=w487, error in=w485) -> (created path=w486:path, error out=w484:errorcluster)  [unwired: 1 in, 1 out]
              }
              frame True {
              }
            }
            n277 = Format Date/Time String(time format string (%c)="%Y%m%d_%H_%M_%S") -> (date/time string=w470:string)  [unwired: 2 in]
            n278 = Index Array(array=w451, index (row)=0 ("禁用的索引 (行)"), index (col)=0 ("禁用的索引 (列)")) -> (element=w448:string)
            n279 = Concatenate Strings(w448, w470, ".JPEG" ("字符串")) -> (w457:string)
            n280 = call "IMAQ Create"("Image Name"="untitled6") -> ("New Image"=w443:T1, "error out"=w442:errorcluster)  [unwired: 4 in]
            n281 = Build Path(base path=w469, name or relative path=w457) -> (appended path=w471:path)
            n282 = call "IMAQ ReadFile 2"("File Path"=path "d:/source.jpg", "error in (no error)"=w442, "Image"=w443) -> ("error out"=w440:errorcluster, "Image Out"=w441:T1)  [unwired: 4 in, 3 out]
            n283 = call-poly "IMAQ Write File 2"("error in (no error)"=w440, "File Path"=w471, "Image"=w441) -> ("error out"=w446:errorcluster, "Image Out (duplicate)"=w447:T1)  [unwired: 7 in]
            n284 = call "IMAQ Dispose"("Image"=w447, "error in (no error)"=w446) -> ("error out"=→"error out 9":errorcluster)  [unwired: 4 in]
          }
          frame #3 {
            n285 = Wait (ms)(milliseconds to wait=u32 2000 ("等待时间（毫秒）")) -> ()  [unwired: 1 out]
          }
          frame #4 {
            w561 = FALSE ("相机识别OK")
            n286 = local write "拍照合格"(w561) -> ()
            n287 = shared-variable "我的电脑\\opc.lvlib\\相机识别OK"(w561) -> ()  [unwired: 1 in, 1 out]
            n288 = shared-variable "我的电脑\\opc.lvlib\\相机识别NG"(w561) -> ()  [unwired: 1 in, 1 out]
            n289 = property on="拍照合格" class="Bool (严格)"("Colors [4]"=cluster{u32, u32}[] [{12369084, 12369084}] ("颜色[4]")) -> ()  [unwired: 2 in, 2 out]
          }
          frame #5 {
            n290 = local write "拍照存储过程"(u8 2 ("拍照存储过程")) -> ()
          }
        }
      }
    }
  }
  n291 = while {
    stop <- FALSE stop-if-true
    n292 = Wait (ms)(milliseconds to wait=u32 100 ("等待时间（毫秒）")) -> ()  [unwired: 1 out]
    n293 = Compound Arithmetic op=OR ("复合运算")("复位", "扫码复位信号", "拍照复位信号") -> (w564:bool)
    n294 = case shown="True" w564 {
      frame False {
      }
      frame True {
        w569 = 0 ("二维码长度")
        w570 = cluster{u32, u32}[] [{12369084, 12369084}] ("颜色[4]")
        w571 = FALSE
        n295 = local write "二维码对应程序号"(w569) -> ()
        n296 = local write "二维码长度"(w569) -> ()
        n297 = local write "二维码"("") -> ()
        n298 = for {
          N: 7 -> [_]
          i -> [w578]
          n299 = for {
            N: 2 -> [_]
            tunnel: w578 -> [w585]
            i -> [w586]
            n300 = Bundle(w585, w586) -> (w584:cluster{i32, i32})  [unwired: 1 in]
            n301 = Initialize Array("", 7 ("维数大小"), 2 ("维数大小")) -> (w582:string[][])
            n302 = property on="扭矩角度表格" class="Tbl (严格)"("Active Cell"=w584, "Cell BG Color"=u32 16448250 ("活动单元格:单元格背景色"), "Value"=w582) -> ()  [unwired: 2 in, 2 out]
          }
        }
        n303 = local write "扫码OK"(w571) -> ()
        n304 = local write "扫码NG"(w571) -> ()
        n305 = Initialize Array("", 7 ("维数大小"), 2 ("维数大小")) -> (w577:string[][])
        n306 = property on="扭矩1合格" class="Bool (严格)"("Colors [4]"=w570) -> ()  [unwired: 2 in, 2 out]
        n307 = property on="扭矩2合格" class="Bool (严格)"("Colors [4]"=w570) -> ()  [unwired: 2 in, 2 out]
        n308 = property on="扭矩3合格" class="Bool (严格)"("Colors [4]"=w570) -> ()  [unwired: 2 in, 2 out]
        n309 = property on="扭矩4合格" class="Bool (严格)"("Colors [4]"=w570) -> ()  [unwired: 2 in, 2 out]
        n310 = property on="扭矩5合格" class="Bool (严格)"("Colors [4]"=w570) -> ()  [unwired: 2 in, 2 out]
        n311 = property on="扭矩6合格" class="Bool (严格)"("Colors [4]"=w570) -> ()  [unwired: 2 in, 2 out]
        n312 = local write "扭矩1合格"(w571) -> ()
        n313 = local write "扭矩2合格"(w571) -> ()
        n314 = local write "扭矩3合格"(w571) -> ()
        n315 = local write "扭矩4合格"(w571) -> ()
        n316 = local write "扭矩5合格"(w571) -> ()
        n317 = local write "扭矩6合格"(w571) -> ()
        n318 = local write "扭矩/角度"(w577) -> ()
        n319 = local write "扭矩7合格"(w571) -> ()
        n320 = property on="扭矩7合格" class="Bool (严格)"("Colors [4]"=w570) -> ()  [unwired: 2 in, 2 out]
      }
    }
  }
  n321 = while {
    shift-right: [w593] -> _
    shift-left: Type."Open" -> [w594]
    shift-right: [w592] -> _
    shift-left: _ -> [w591]
    tunnel: "错误输入（无错误）" -> [w590]
    tunnel: [w589] -> w10
    stop <- FALSE stop-if-true
    n322 = case shown="\"Read\"" w594 {
      tunnel: [w597 Type."Loop" Type."Read" w643 Type."Loop" Type."Exit" Type."Write"] -> w593
      tunnel: [w595 w604 w608 w647 w715 w722 w726] -> w592
      tunnel: w591 -> [w595 _ w612 w644 w718 w722 w726]
      tunnel: w590 -> [w596 w607 w611 w650 w719 w721 w725]
      tunnel: [w596 w606 w610 w648 w717 w720 w725] -> w589
      frame "Init", Default {
        n323 = Unbundle By Name(w596) -> ("status"=w598:bool)
        n324 = case shown="False" w598 {
          tunnel: [Type."Loop" Type."Exit"] -> w597
          frame False {
          }
          frame True {
          }
        }
      }
      frame "Open" {
        n325 = TCP Open Connection(address="192.168.1.32" ("地址"), remote port or service name=9004 ("超时毫秒(60000)"), timeout ms (60000)=1000 ("超时毫秒(60000)"), error in (no error)=w607) -> (connection ID=w604:refnum<k5>, error out=w606:errorcluster)  [unwired: 1 in]
      }
      frame "Write" {
        n326 = case shown="False" "开始扫码" {
          tunnel: w612 -> [w615 w638]
          tunnel: w611 -> [w617 w637]
          tunnel: [w616 w636] -> w610
          tunnel: [w614 w631] -> w608
          frame False {
            n327 = case shown="False" "扫码复位" {
              tunnel: w617 -> [w620 w626]
              tunnel: [w620 w625] -> w616
              tunnel: w615 -> [w619 w624]
              tunnel: [w619 w623] -> w614
              frame False {
              }
              frame True {
                w621 = FALSE ("扫码NG")
                n328 = local write "二维码"("") -> ()
                n329 = local write "扫码NG"(w621) -> ()
                n330 = local write "扫码OK"(w621) -> ()
                n331 = Concatenate Strings("LOFF", "\r") -> (w630:string)
                n332 = TCP Write(connection ID=w624, data in=w630, error in (no error)=w626, 9:100 ("超时毫秒(25000)")) -> (connection ID out=w623:refnum<k5>, error out=w625:errorcluster)  [unwired: 1 out]
              }
            }
          }
          frame True {
            n333 = Concatenate Strings("LON", "\r") -> (w632:string)
            n334 = TCP Write(connection ID=w638, data in=w632, error in (no error)=w637, 9:100 ("超时毫秒(25000)")) -> (connection ID out=w631:refnum<k5>, error out=w636:errorcluster)  [unwired: 1 out]
          }
        }
      }
      frame "Read" {
        n335 = TCP Read(connection ID=w644, bytes to read=50 ("读取的字节"), error in (no error)=w650, 7:T11."Immediate" ("模式（标准）"), 9:100 ("超时毫秒(25000)")) -> (connection ID out=w647:refnum<k5>, data out=w642:string, error out=w648:errorcluster)
        n336 = String Length(string=w642) -> (length=w641:i32)
        n337 = Greater?(x=w641, y=20) -> (0:w639:bool)
        n338 = case shown="True" w639 {
          tunnel: w642 -> [w654 _]
          tunnel: [Type."Loop" Type."Loop"] -> w643
          frame True {
            n339 = local read "产品参数列表（点击表格内任意位置，即可选中所对应产品）"() -> (w660:string[][])
            n340 = String Length(string=w654) -> (length=w653:i32)
            n341 = Decrement(x=w653) -> (x-1=w652:i32)
            n342 = String Subset "截取字符串"(string=w654, offset (0)=0 ("偏移量(0)"), length (rest)=w652) -> (substring=w656:string)
            n343 = local read "已选产品"() -> (w662:string[][])
            n344 = local write "二维码"(w656) -> ()
            n345 = Index Array(array=w662, index (row)=0 ("禁用的索引 (行)"), index (col)=1 ("禁用的索引 (列)")) -> (element=w675:string)
            n346 = Index Array(array=w662, index (row)=0 ("禁用的索引 (行)"), index (col)=2 ("禁用的索引 (列)")) -> (element=w669:string)
            n347 = String Subset(string=w656, length (rest)=6 ("长度（剩余）")) -> (substring=w658:string)  [unwired: 1 in]
            n348 = Decimal String To Number(string=w669) -> (number=w668:i32)  [unwired: 2 in, 1 out]
            n349 = String Length(string=w656) -> (length=w651:i32)
            "二维码长度" <- w651
            n350 = String Subset(string=w675, length (rest)=5 ("长度（剩余）")) -> (substring=w673:string)  [unwired: 1 in]
            n351 = String Subset(string=w656, length (rest)=5 ("长度（剩余）")) -> (substring=w655:string)  [unwired: 1 in]
            n352 = Search and Replace String(input string=w654, search string=w673) -> (number of replacements=w667:i32)  [unwired: 6 in, 3 out]
            n353 = for {
              N: 50 -> [_]
              tunnel: w660 -> [w685]
              tunnel: w658 -> [w691]
              tunnel: w655 -> [w684]
              i -> [w687]
              n354 = Index Array(array=w685, index (row)=w687, index (col)=1 ("禁用的索引 (列)")) -> (element=w692:string)
              n355 = Increment(x=w687) -> (x+1=w688:i32)
              n356 = Search and Replace String(input string=w692, search string=w691) -> (number of replacements=w682:i32)  [unwired: 6 in, 3 out]
              n357 = Equal?(x=w687, y=49) -> (x = y?=w681:bool)
              n358 = Equal?(x=w682, y=0) -> (x = y?=w680:bool)
              n359 = Equal?(x=w682, y=1) -> (x = y?=w689:bool)
              n360 = case shown="True" w689 {
                tunnel: w688 -> [_ w707]
                frame False {
                }
                frame True {
                  "二维码对应程序号" <- w707
                }
              }
              n361 = And(x=w680, y=w681) -> (x .and. y?=w679:bool)
              n362 = case shown="True" w679 {
                tunnel: w685 -> [_ w695]
                tunnel: w684 -> [_ w694]
                frame False {
                }
                frame True {
                  n363 = for {
                    N: 50 -> [_]
                    tunnel: w695 -> [w705]
                    tunnel: w694 -> [w700]
                    i -> [w698]
                    n364 = Index Array(array=w705, index (row)=w698, index (col)=1 ("禁用的索引 (列)")) -> (element=w701:string)
                    n365 = Search and Replace String(input string=w701, search string=w700) -> (number of replacements=w702:i32)  [unwired: 6 in, 3 out]
                    n366 = Increment(x=w698) -> (x+1=w697:i32)
                    n367 = Equal?(x=w702, y=1) -> (x = y?=w699:bool)
                    n368 = case shown="True" w699 {
                      tunnel: w697 -> [_ w706]
                      frame False {
                      }
                      frame True {
                        n369 = local write "二维码对应程序号"(w706) -> ()
                      }
                    }
                  }
                }
              }
            }
            n370 = Equal?(x=w651, y=w668) -> (x = y?=w666:bool)
            n371 = Equal?(x=w667, y=1) -> (x = y?=w665:bool)
            n372 = And(x=w665, y=w666) -> (x .and. y?=w663:bool)
            n373 = case shown="True" w663 {
              frame False {
                n374 = flat-sequence {
                  frame #0 {
                    "扫码NG" <- TRUE
                  }
                  frame #1 {
                    n375 = Wait (ms)(milliseconds to wait=u32 2000 ("等待时间（毫秒）")) -> ()  [unwired: 1 out]
                  }
                  frame #2 {
                    w710 = FALSE ("扫码OK")
                    n376 = local write "扫码NG"(w710) -> ()
                    n377 = local write "扫码OK"(w710) -> ()
                  }
                }
              }
              frame True {
                n378 = flat-sequence {
                  frame #0 {
                    "扫码OK" <- TRUE ("扫码OK")
                  }
                  frame #1 {
                    n379 = Wait (ms)(milliseconds to wait=u32 2000 ("等待时间（毫秒）")) -> ()  [unwired: 1 out]
                  }
                  frame #2 {
                    w713 = FALSE ("扫码OK")
                    n380 = local write "扫码NG"(w713) -> ()
                    n381 = local write "扫码OK"(w713) -> ()
                  }
                }
              }
            }
          }
          frame False {
          }
        }
      }
      frame "Close" {
        n382 = TCP Close Connection(connection ID=w718, error in (no error)=w719) -> (connection ID out=w715:refnum<k5>, error out=w717:errorcluster)  [unwired: 1 in]
      }
      frame "Exit" {
        n383 = TCP Close Connection(connection ID=w722, error in (no error)=w721) -> (error out=w720:errorcluster)  [unwired: 1 in, 1 out]
      }
      frame "Loop" {
      }
    }
  }
  "错误输出" <- w10
  n384 = while {
    shift-right: [w733] -> _
    shift-left: Type."Open" -> [w734]
    shift-right: [w732] -> _
    shift-left: _ -> [w731]
    tunnel: "错误输入（无错误） 2" -> [w730]
    tunnel: [w729] -> w9
    stop <- FALSE stop-if-true
    n385 = case shown="\"Read\"" w734 {
      tunnel: [w737 Type."Loop" w751 w770 Type."Loop" Type."Exit" w825] -> w733
      tunnel: [w735 w744 w750 w774 w808 w815 w827] -> w732
      tunnel: w731 -> [w735 _ w756 w773 w811 w815 w827]
      tunnel: w730 -> [w736 w747 w755 w776 w812 w814 w826]
      tunnel: [w736 w746 w754 w775 w810 w813 w826] -> w729
      frame "Init", Default {
        n386 = Unbundle By Name(w736) -> ("status"=w738:bool)
        n387 = case shown="True" w738 {
          tunnel: [Type."Loop" Type."Exit"] -> w737
          frame False {
          }
          frame True {
          }
        }
      }
      frame "Open" {
        n388 = TCP Open Connection(address="192.168.1.56" ("地址"), remote port or service name=50000 ("超时毫秒(60000)"), timeout ms (60000)=1000 ("超时毫秒(60000)"), error in (no error)=w747) -> (connection ID=w744:refnum<k5>, error out=w746:errorcluster)  [unwired: 1 in]
      }
      frame "Write" {
        n389 = flat-sequence {
          tunnel: w756 -> [w763]
          tunnel: w755 -> [w762]
          tunnel: [w761] -> w753
          tunnel: [w757] -> w748
          tunnel: w753 -> [w766]
          tunnel: [w766] -> w752
          tunnel: [w765] -> w749
          tunnel: w748 -> [w765]
          tunnel: [w769] -> w754
          tunnel: w752 -> [w769]
          tunnel: [Type."Read"] -> w751
          tunnel: [w767] -> w750
          tunnel: w749 -> [w767]
          frame #0 {
            n390 = call "字符串转十六进制.vi"("字符串"="FD 01 00 92 00 FE") -> ("十六进制整型字符串"=w759:string)  [unwired: 10 in]
            n391 = TCP Write(connection ID=w763, data in=w759, error in (no error)=w762, 9:100 ("超时毫秒(25000)")) -> (connection ID out=w757:refnum<k5>, error out=w761:errorcluster)  [unwired: 1 out]
          }
          frame #1 {
            n392 = Wait (ms)(milliseconds to wait=u32 500 ("等待时间（毫秒）")) -> ()  [unwired: 1 out]
          }
          frame #2 {
          }
        }
      }
      frame "Read" {
        n393 = flat-sequence {
          tunnel: w776 -> [w784]
          tunnel: w773 -> [w777]
          tunnel: [w782] -> w772
          tunnel: [w780] -> w771
          tunnel: [w806] -> w774
          tunnel: [w807] -> w775
          tunnel: w772 -> [w807]
          tunnel: w771 -> [w806]
          tunnel: [Type."Loop"] -> w770
          frame #0 {
            n394 = TCP Read(connection ID=w777, bytes to read=500 ("读取的字节"), error in (no error)=w784, 7:T11."Standard" ("模式（标准）"), 9:100 ("超时毫秒(25000)")) -> (connection ID out=w780:refnum<k5>, data out=w781:string, error out=w782:errorcluster)
            n395 = Empty String/Path?(string/path=w781) -> (empty?=w785:bool)
            n396 = case shown="False" w785 {
              tunnel: w781 -> [w800 _]
              frame False {
                n397 = String Subset(string=w800, offset (0)=45 ("偏移量(0)"), length (rest)=4 ("长度（剩余）")) -> (substring=w799:string)
                n398 = String Subset(string=w800, offset (0)=68 ("偏移量(0)"), length (rest)=4 ("长度（剩余）")) -> (substring=w798:string)
                n399 = call "十六进制字符串至普通字符串转换(个人编写).vi"("十六进制字符串"=w799) -> ("普通字符串"=w797:string)
                n400 = call "十六进制字符串至普通字符串转换(个人编写).vi"("十六进制字符串"=w798) -> ("普通字符串"=w789:string)
                n401 = Decimal String To Number(string=w797) -> (number=w796:i32)  [unwired: 2 in, 1 out]
                n402 = Decimal String To Number(string=w789) -> (number=w790:i32)  [unwired: 2 in, 1 out]
                n403 = Divide(x=w790, y=10) -> (x/y=w788:dbl)
                n404 = Divide(x=w796, y=10000) -> (x/y=w794:dbl)
                n405 = Number To Fractional String(number=w788, precision (6)=i16 2 ("精度(6)")) -> (F-format string=→"角度字符串":string)  [unwired: 2 in]
                n406 = Number To Fractional String(number=w794, precision (6)=i16 2 ("精度(6)")) -> (F-format string=→"扭矩字符串":string)  [unwired: 2 in]
                "读到的数据" <- w800
              }
              frame True {
              }
            }
          }
          frame #1 {
          }
        }
      }
      frame "Close" {
        n407 = TCP Close Connection(connection ID=w811, error in (no error)=w812) -> (connection ID out=w808:refnum<k5>, error out=w810:errorcluster)  [unwired: 1 in]
      }
      frame "Exit" {
        (unwired) TRUE
        n408 = TCP Close Connection(connection ID=w815, error in (no error)=w814) -> (error out=w813:errorcluster)  [unwired: 1 in, 1 out]
      }
      frame "Loop" {
        n409 = Compound Arithmetic op=OR ("复合运算")("螺栓0扭矩读取", "螺栓1扭矩读取", "螺栓2扭矩读取", "螺栓3扭矩读取", "螺栓4扭矩读取", "螺栓5扭矩读取", "螺栓6扭矩读取") -> (w824:bool)
        n410 = case shown="False" w824 {
          tunnel: [Type."Read" Type."Write"] -> w825
          frame False {
          }
          frame True {
          }
        }
      }
    }
    n411 = Wait (ms)(milliseconds to wait=u32 1 ("等待时间（毫秒）")) -> ()  [unwired: 1 out]
  }
  "错误输出 2" <- w9
  n412 = while {
    stop <- FALSE stop-if-true
    n413 = Wait (ms)(milliseconds to wait=u32 100 ("等待时间（毫秒）")) -> ()  [unwired: 1 out]
    n414 = case shown="False" "用户退出" {
      frame False {
      }
      frame True {
      }
    }
    n415 = case shown="0, 默认" "登录过程" {
      tunnel: "用户登录" -> [w835 _ w944]
      frame 0, Default {
        n416 = case shown="False" w835 {
          frame False {
          }
          frame True {
            n417 = local write "登录过程"(1.0 ("登录过程")) -> ()
          }
        }
      }
      frame 1 {
        n418 = Search and Replace String(input string="密码", search string="1111" ("搜索字符串")) -> (number of replacements=w844:i32)  [unwired: 6 in, 3 out]
        n419 = Search and Replace String(input string="用户名", search string="admin" ("替换字符串(\"\")")) -> (number of replacements=w839:i32)  [unwired: 6 in, 3 out]
        n420 = Equal?(x=w839, y=1) -> (x = y?=w843:bool)
        n421 = Equal?(x=w844, y=1) -> (x = y?=w842:bool)
        n422 = And(x=w843, y=w842) -> (x .and. y?=w841:bool)
        n423 = case shown="True" w841 {
          frame False {
            n424 = flat-sequence {
              frame #0 {
                w848 = ""
                n425 = local write "用户名"(w848) -> ()
                n426 = local write "密码"(w848) -> ()
                n427 = One Button Dialog(message="用户名或密码错误" ("消息")) -> ()  [unwired: 1 in, 1 out]
              }
              frame #1 {
                n428 = local write "登录过程"(2.0 ("登录过程")) -> ()
              }
            }
          }
          frame True {
            n429 = flat-sequence {
              tunnel: [w872] -> w854
              tunnel: [w871] -> w853
              tunnel: w854 -> [w908]
              tunnel: w853 -> [w907]
              tunnel: [w905] -> w852
              tunnel: [w906] -> w851
              tunnel: w852 -> [w942]
              tunnel: w851 -> [w941]
              frame #0 {
              }
              frame #1 {
                n430 = for {
                  N: 100 -> [_]
                  i -> [w861]
                  n431 = Quotient & Remainder(x=w861, y=2) -> (x-y*floor(x/y)=w859:i32)  [unwired: 1 out]
                  n432 = Equal To 0?(x=w859) -> (x = 0?=w858:bool)
                  n433 = case shown="True" w858 {
                    tunnel: [u32 12369084 ("活动单元格:单元格背景色") u32 16448250 ("活动单元格:单元格背景色")] -> w856
                    frame False {
                    }
                    frame True {
                    }
                  }
                  n434 = for {
                    N: 15 -> [_]
                    tunnel: w861 -> [w867]
                    tunnel: w856 -> [w865]
                    i -> [w866]
                    n435 = Bundle(w867, w866) -> (w864:cluster{i32, i32})  [unwired: 1 in]
                    n436 = property on="产品参数列表（点击表格内任意位置，即可选中所对应产品）" class="Tbl (严格)"("Active Cell"=w864, "Cell BG Color"=w865) -> ()  [unwired: 2 in, 2 out]
                  }
                }
              }
              frame #2 {
              }
              frame #3 {
              }
              frame #4 {
                n437 = property on="产品参数列表（点击表格内任意位置，即可选中所对应产品）" class="Tbl (严格)"() -> ("Column Headers[]"=w877:string[])  [unwired: 2 in, 2 out]
                n438 = property on="作业员列表" class="Tbl (严格)"("Active Cell"=T2 {"Row"=-2, "Column"=-2} ("活动单元格:活动单元格"), "Value"=string[][] [["", "", "", ""], ["", "", "", ""], ["", "", "", ""], ["", "", "", ""], ["", "", "", ""], ["", "", "", ""], ["", "", "", ""], ["", "", "", ""], ["", "", "", ""], ["", "", "", ""], ["", "", "", ""], ["", "", "", ""], ["", "", "", ""], ["", "", "", ""], ["", "", "", ""], ["", "", "", ""], ["", "", "", ""], ["", "", "", ""], ["", "", "", ""], ["", "", "", ""], ["", "", "", ""], ["", "", "", ""], ["", "", "", ""], ["", "", "", ""], ["", "", "", ""], ["", "", "", ""], ["", "", "", ""], ["", "", "", ""], ["", "", "", ""], ["", "", "", ""], ["", "", "", ""], ["", "", "", ""], ["", "", "", ""], ["", "", "", ""], ["", "", "", ""], ["", "", "", ""], ["", "", "", ""], ["", "", "", ""], ["", "", "", ""], ["", "", "", ""], ["", "", "", ""], ["", "", "", ""], ["", "", "", ""], ["", "", "", ""], ["", "", "", ""], ["", "", "", ""], ["", "", "", ""], ["", "", "", ""], ["", "", "", ""], ["", "", "", ""], ["", "", "", ""], ["", "", "", ""], ["", "", "", ""], ["", "", "", ""], ["", "", "", ""], ["", "", "", ""], ["", "", "", ""], ["", "", "", ""], ["", "", "", ""], ["", "", "", ""], ["", "", "", ""], ["", "", "", ""], ["", "", "", ""], ["", "", "", ""], ["", "", "", ""], ["", "", "", ""], ["", "", "", ""], ["", "", "", ""], ["", "", "", ""], ["", "", "", ""], ["", "", "", ""], ["", "", "", ""], ["", "", "", ""], ["", "", "", "0"]] ("表格控件")) -> ()  [unwired: 2 in, 2 out]
                n439 = Array Size(array=w877) -> (size(s)=w875:i32)
                n440 = Initialize Array("", 100 ("维数大小"), w875) -> (w873:string[][])
                n441 = call <vilib>:"Open Config Data.vi"("create file if necessary (T)"=TRUE, "configuration file path"=path "D:/Test/Setup.ini") -> ("error out"=w880:errorcluster, "refnum"=w878:T4)  [unwired: 7 in, 1 out]
                n442 = for {
                  N: w875 -> [_]
                  tunnel: w878 -> [w889]
                  tunnel: w880 -> [w888]
                  tunnel: w877 -> [w887]
                  tunnel: [w885] -> w872
                  tunnel: [w884] -> w871
                  shift-right: [w881] -> _
                  shift-left: w873 -> [w882]
                  i -> [w883]
                  n443 = Index Array(array=w887, index=w883) -> (element=w886:string)
                  n444 = for {
                    N: 100 -> [_]
                    tunnel: w889 -> [w904]
                    tunnel: [w902] -> w885
                    tunnel: w888 -> [w901]
                    tunnel: [w900] -> w884
                    tunnel: w886 -> [w896]
                    tunnel: w883 -> [_]
                    tunnel: w883 -> [w894]
                    shift-right: [w891] -> w881
                    shift-left: w882 -> [w892]
                    i -> [w895]
                    n445 = Increment(x=w895) -> (x+1=w899:i32)
                    n446 = Number To Decimal String(number=w899) -> (decimal integer string=w898:string)  [unwired: 1 in]
                    n447 = Concatenate Strings(w896, w898) -> (w897:string)
                    n448 = call-poly <vilib>:"Read Key.vi"("section"="Setup", "error in (no error)"=w901, "key"=w897, "refnum"=w904) -> ("error out"=w900:errorcluster, "value"=w893:string, "refnum out"=w902:T4)  [unwired: 4 in, 1 out]
                    n449 = Replace Array Subset "替换数组子集"(array=w892, new element=w893, index (row)=w895, index (col)=w894) -> (w891:string[][])
                    n450 = local write "产品参数列表（点击表格内任意位置，即可选中所对应产品）"(w891) -> ()
                  }
                }
              }
              frame #5 {
                n451 = for {
                  N: 10 -> [_]
                  tunnel: w908 -> [w940]
                  tunnel: [w938] -> w912
                  tunnel: w907 -> [w937]
                  tunnel: [w936] -> w911
                  i -> [w930]
                  n452 = Increment(x=w930) -> (x+1=w934:i32)
                  n453 = Number To Decimal String(number=w934) -> (decimal integer string=w933:string)  [unwired: 1 in]
                  n454 = Concatenate Strings("作业员编码" ("字符串"), w933) -> (w932:string)
                  n455 = local read "作业员列表"() -> (w928:string[][])
                  n456 = call-poly <vilib>:"Read Key.vi"("section"="Setup", "error in (no error)"=w937, "key"=w932, "refnum"=w940) -> ("error out"=w936:errorcluster, "value"=w931:string, "refnum out"=w938:T4)  [unwired: 4 in, 1 out]
                  n457 = Replace Array Subset(array=w928, new element=w931, index (row)=w930, index (col)=0 ("索引 (列)")) -> (w927:string[][])
                  n458 = local write "作业员列表"(w927) -> ()
                }
                n459 = for {
                  N: 10 -> [_]
                  tunnel: w912 -> [w926]
                  tunnel: [w924] -> w906
                  tunnel: w911 -> [w923]
                  tunnel: [w915] -> w905
                  i -> [w917]
                  n460 = Increment(x=w917) -> (x+1=w921:i32)
                  n461 = Number To Decimal String(number=w921) -> (decimal integer string=w920:string)  [unwired: 1 in]
                  n462 = Concatenate Strings("作业员姓名" ("字符串"), w920) -> (w919:string)
                  n463 = local read "作业员列表"() -> (w913:string[][])
                  n464 = call-poly <vilib>:"Read Key.vi"("section"="Setup", "error in (no error)"=w923, "key"=w919, "refnum"=w926) -> ("error out"=w915:errorcluster, "value"=w918:string, "refnum out"=w924:T4)  [unwired: 4 in, 1 out]
                  n465 = Replace Array Subset(array=w913, new element=w918, index (row)=w917, index (col)=1 ("索引 (列)")) -> (w914:string[][])
                  n466 = local write "作业员列表"(w914) -> ()
                }
              }
              frame #6 {
                n467 = call <vilib>:"Close Config Data.vi"("error in (no error)"=w942, "refnum"=w941) -> ()  [unwired: 8 in, 2 out]
              }
              frame #7 {
                n468 = local write "登录过程"(2.0 ("登录过程")) -> ()
              }
            }
          }
        }
      }
      frame 2 {
        n469 = case shown="False" w944 {
          frame False {
            n470 = local write "登录过程"(0.0 ("登录过程")) -> ()
          }
          frame True {
          }
        }
      }
    }
  }
  n471 = flat-sequence {
    frame #0 {
    }
    frame #1 {
    }
    frame #2 {
      w953 = 7
      n472 = for {
        N: 7 -> [_]
        i -> [w964]
        n473 = for {
          N: 2 -> [_]
          tunnel: w964 -> [w971]
          i -> [w972]
          n474 = Bundle(w971, w972) -> (w970:cluster{i32, i32})  [unwired: 1 in]
          n475 = Initialize Array("", 7 ("维数大小"), 2 ("维数大小")) -> (w968:string[][])
          n476 = property on="扭矩角度表格" class="Tbl (严格)"("Active Cell"=w970, "Cell BG Color"=u32 16448250 ("活动单元格:单元格背景色"), "Value"=w968) -> ()  [unwired: 2 in, 2 out]
        }
      }
      n477 = Initialize Array("", 1 ("维数大小"), 9 ("维数大小")) -> (w959:string[][])
      n478 = Initialize Array("", 50 ("维数大小"), 9 ("维数大小")) -> (w960:string[][])
      n479 = Initialize Array("", w953) -> (w951:string[])
      n480 = local write "产品参数列表（点击表格内任意位置，即可选中所对应产品）"(w960) -> ()
      n481 = local write "已选产品"(w959) -> ()
      n482 = for {
        N: w953 -> [_]
        shift-right: [w978] -> _
        shift-left: 0.0 -> [w979]
        shift-right: [w975] -> w949
        shift-left: w951 -> [w976]
        i -> [w980]
        n483 = Increment(x=w979) -> (x+1=w978:dbl)
        n484 = Number To Decimal String(number=w978, width (-)=i16 3 ("宽度(-)")) -> (decimal integer string=w977:string)
        n485 = Replace Array Subset(array=w976, new element=w977, index=w980) -> (w975:string[])
      }
      n486 = local write "二维码对应程序号"(i16 0 ("宽度(-)")) -> ()
      n487 = Build Array("扭矩（N.m)", "角度（°)") -> (w955:string[])
      n488 = property on="扭矩角度表格" class="Tbl (严格)"("Row Headers[]"=w949, "Column Headers[]"=w955) -> ()  [unwired: 2 in, 2 out]
    }
    frame #3 {
      w981 = cluster{u32, u32}[] [{12369084, 12369084}] ("颜色[4]")
      w984 = FALSE
      w1045 = ""
      w1046 = u32 345 ("大小:高度")
      w1056 = 99
      w1058 = T12 {"Width"=180, "Height"=180} ("按钮大小")
      w1059 = 999
      w1067 = 999
      w1044 = u32 25 ("标签.字体:字号")
      n489 = call "数据查询.vi"() -> ("今日合格数"=w1009:i32, "今日总数"=w1010:i32, "Data"=w1011:string[][])  [unwired: 9 in]
      n490 = local write "产品型号选择"(i16 1 ("产品型号选择")) -> ()
      n491 = local read "已选产品"() -> (w989:string[][])
      n492 = property on="扭矩1合格" class="Bool (严格)"("Button Size"=w1058) -> ()  [unwired: 2 in, 2 out]
      n493 = property on="扭矩2合格" class="Bool (严格)"("Button Size"=w1058) -> ()  [unwired: 2 in, 2 out]
      n494 = property on="扭矩3合格" class="Bool (严格)"("Button Size"=w1058) -> ()  [unwired: 2 in, 2 out]
      n495 = property on="扭矩4合格" class="Bool (严格)"("Button Size"=w1058) -> ()  [unwired: 2 in, 2 out]
      n496 = local write "表格"(w1011) -> ()
      n497 = for {
        N: 2 -> [_]
        i -> [w1111]
        n498 = for {
          N: 4 -> [_]
          tunnel: w1111 -> [w1114]
          i -> [w1115]
          n499 = Decrement(x=w1114) -> (x-1=w1113:i32)
          n500 = Bundle(cluster="活动单元格:活动单元格 3", "Row"=w1113, "Column"=w1115) -> (w1116:T2)
          n501 = property on="已选产品" class="Tbl (严格)"("Active Cell"=w1116, "CellFontSize"=u32 25 ("活动单元格:单元格字体:字号")) -> ()  [unwired: 2 in, 2 out]
        }
      }
      n502 = property on="作业员列表" class="Tbl (严格)"("Height"=w1046) -> ()  [unwired: 2 in, 2 out]
      n503 = property on="产品参数列表（点击表格内任意位置，即可选中所对应产品）" class="Tbl (严格)"("Height"=w1046) -> ()  [unwired: 2 in, 2 out]
      n504 = for {
        N: 99 -> [_]
        i -> [w1119]
        n505 = for {
          N: 3 -> [_]
          tunnel: w1119 -> [w1124]
          i -> [w1122]
          n506 = Decrement(x=w1124) -> (x-1=w1123:i32)
          n507 = Decrement(x=w1122) -> (x-1=w1121:i32)
          n508 = Bundle(cluster="活动单元格:活动单元格 5", "Row"=w1123, "Column"=w1121) -> (w1125:T2)
          n509 = property on="作业员列表" class="Tbl (严格)"("Active Cell"=w1125, "CellFontSize"=u32 25 ("活动单元格:单元格字体:字号")) -> ()  [unwired: 2 in, 2 out]
        }
      }
      n510 = property on="二维码" class="Str"("Label.FontSize"=w1044) -> ()  [unwired: 2 in, 2 out]
      n511 = property on="作业员列表" class="Tbl (严格)"("Label.FontSize"=w1044) -> ()  [unwired: 2 in, 2 out]
      n512 = property on="扭矩/角度" class="Arr (严格)"("Label.FontSize"=w1044) -> ()  [unwired: 2 in, 2 out]
      n513 = property on="用户名" class="Str"("Text.FontSize"=w1044, "Text.Text"=w1045) -> ()  [unwired: 2 in, 2 out]
      n514 = property on="密码" class="Str"("Text.FontSize"=w1044, "Text.Text"=w1045) -> ()  [unwired: 2 in, 2 out]
      n515 = property on="今日合格" class="Str"("Text.FontSize"=w1044, "Label.FontSize"=w1044) -> ()  [unwired: 2 in, 2 out]
      n516 = property on="作业员 Operator" class="Ring (严格)"("Label.FontSize"=w1044) -> ()  [unwired: 2 in, 2 out]
      n517 = property on="扭矩1合格" class="Bool (严格)"("Label.FontSize"=w1044) -> ()  [unwired: 2 in, 2 out]
      n518 = property on="扭矩3合格" class="Bool (严格)"("Label.FontSize"=w1044) -> ()  [unwired: 2 in, 2 out]
      n519 = property on="产品参数列表（点击表格内任意位置，即可选中所对应产品）" class="Tbl (严格)"("Label.FontSize"=w1044) -> ()  [unwired: 2 in, 2 out]
      n520 = property on="扭矩2合格" class="Bool (严格)"("Label.FontSize"=w1044) -> ()  [unwired: 2 in, 2 out]
      n521 = property on="今日总数" class="Str"("Text.FontSize"=w1044, "Label.FontSize"=w1044) -> ()  [unwired: 2 in, 2 out]
      n522 = property on="待拧紧前识别图像" class="ImageControl"("Label.FontSize"=w1044) -> ()  [unwired: 2 in, 2 out]
      n523 = property on="扭矩4合格" class="Bool (严格)"("Label.FontSize"=w1044) -> ()  [unwired: 2 in, 2 out]
      n524 = for {
        N: 1000 -> [_]
        i -> [w1128]
        n525 = for {
          N: 7 -> [_]
          tunnel: w1128 -> [w1133]
          i -> [w1131]
          n526 = Decrement(x=w1133) -> (x-1=w1132:i32)
          n527 = Decrement(x=w1131) -> (x-1=w1130:i32)
          n528 = Bundle(cluster="活动单元格:活动单元格 4", "Row"=w1132, "Column"=w1130) -> (w1134:T2)
          n529 = property on="产品参数列表（点击表格内任意位置，即可选中所对应产品）" class="Tbl (严格)"("Active Cell"=w1134, "CellFontSize"=u32 25 ("活动单元格:单元格字体:字号")) -> ()  [unwired: 2 in, 2 out]
        }
      }
      n530 = Initialize Array("", 7 ("维数大小"), 2 ("维数大小")) -> (→"扭矩/角度":string[][])
      n531 = Initialize Array("", w1056) -> (w1054:string[])
      n532 = Initialize Array("", w1059) -> (w1061:string[])
      n533 = Initialize Array("", w1067) -> (w1065:string[])
      n534 = property on="扭矩1合格" class="Bool (严格)"("Colors [4]"=w981) -> ()  [unwired: 2 in, 2 out]
      n535 = property on="扭矩2合格" class="Bool (严格)"("Colors [4]"=w981) -> ()  [unwired: 2 in, 2 out]
      n536 = property on="扭矩3合格" class="Bool (严格)"("Colors [4]"=w981) -> ()  [unwired: 2 in, 2 out]
      n537 = property on="扭矩5合格" class="Bool (严格)"("Colors [4]"=w981) -> ()  [unwired: 2 in, 2 out]
      n538 = property on="扭矩4合格" class="Bool (严格)"("Colors [4]"=w981) -> ()  [unwired: 2 in, 2 out]
      n539 = property on="扭矩6合格" class="Bool (严格)"("Colors [4]"=w981) -> ()  [unwired: 2 in, 2 out]
      n540 = Number To Decimal String(number=w1010) -> (decimal integer string=w1008:string)  [unwired: 1 in]
      n541 = Number To Decimal String(number=w1009) -> (decimal integer string=w1007:string)  [unwired: 1 in]
      n542 = call <vilib>:"Open Config Data.vi"("create file if necessary (T)"=TRUE, "configuration file path"=path "D:/setup.ini") -> ("error out"=w1005:errorcluster, "refnum"=w1006:T4)  [unwired: 7 in, 1 out]
      n543 = call <vilib>:"Open Config Data.vi"("create file if necessary (T)"=TRUE, "configuration file path"=path "D:/setup.ini") -> ("error out"=w994:errorcluster, "refnum"=w993:T4)  [unwired: 7 in, 1 out]
      n544 = Replace Array Subset(array=w989, new element="1", index (row)=0 ("索引 (行)"), index (col)=8 ("禁用的索引 (列)")) -> (w990:string[][])
      n545 = local write "今日总数"(w1008) -> ()
      n546 = local write "今日合格"(w1007) -> ()
      n547 = property on="扭矩7合格" class="Bool (严格)"("Colors [4]"=w981) -> ()  [unwired: 2 in, 2 out]
      n548 = local write "已选产品"(w990) -> ()
      n549 = for {
        N: w1056 -> [_]
        shift-right: [w1141] -> _
        shift-left: 0.0 -> [w1142]
        shift-right: [w1138] -> w1053
        shift-left: w1054 -> [w1139]
        i -> [w1143]
        n550 = Increment(x=w1142) -> (x+1=w1141:dbl)
        n551 = Number To Decimal String(number=w1141, width (-)=i16 2 ("宽度(-)")) -> (decimal integer string=w1140:string)
        n552 = Replace Array Subset(array=w1139, new element=w1140, index=w1143) -> (w1138:string[])
      }
      n553 = for {
        N: w1059 -> [_]
        shift-right: [w1148] -> _
        shift-left: 0.0 -> [w1149]
        shift-right: [w1145] -> w1051
        shift-left: w1061 -> [w1146]
        i -> [w1150]
        n554 = Increment(x=w1149) -> (x+1=w1148:dbl)
        n555 = Number To Decimal String(number=w1148, width (-)=i16 3 ("宽度(-)")) -> (decimal integer string=w1147:string)
        n556 = Replace Array Subset(array=w1146, new element=w1147, index=w1150) -> (w1145:string[])
      }
      n557 = for {
        N: 2 -> [_]
        tunnel: w1006 -> [w1074]
        tunnel: [w1071] -> w1002
        tunnel: w1005 -> [w1073]
        tunnel: [w1070] -> w1001
        i -> [w1069]
        n558 = for {
          N: 50 -> [_]
          tunnel: w1074 -> [w1089]
          tunnel: w1073 -> [w1088]
          tunnel: [w1079] -> w1071
          tunnel: [w1078] -> w1070
          tunnel: w1069 -> [w1077]
          i -> [w1075]
          n559 = property on="作业员列表" class="Tbl (严格)"() -> ("Column Headers[]"=w1086:string[], "Value"=w1082:string[][])  [unwired: 2 in, 2 out]
          n560 = Index Array(array=w1086, index=w1077) -> (element=w1085:string)
          n561 = Number To Decimal String(number=w1075) -> (decimal integer string=w1084:string)  [unwired: 1 in]
          n562 = Concatenate Strings(w1085, w1084) -> (w1083:string)
          n563 = Decrement(x=w1075) -> (x-1=w1076:i32)
          n564 = call-poly <vilib>:"Read Key.vi"("section"="Setup", "error in (no error)"=w1088, "key"=w1083, "refnum"=w1089) -> ("error out"=w1078:errorcluster, "value"=w1080:string, "refnum out"=w1079:T4)  [unwired: 4 in, 1 out]
          n565 = Replace Array Subset(array=w1082, new element=w1080, index (row)=w1076, index (col)=w1077) -> (w1081:string[][])
          n566 = property on="作业员列表" class="Tbl (严格)"("Value"=w1081) -> ()  [unwired: 2 in, 2 out]
        }
      }
      n567 = for {
        N: 9 -> [_]
        tunnel: w993 -> [w1095]
        tunnel: [w1092] -> w997
        tunnel: w994 -> [w1094]
        tunnel: [w1091] -> w998
        i -> [w1090]
        n568 = for {
          N: 50 -> [_]
          tunnel: w1095 -> [w1110]
          tunnel: w1094 -> [w1109]
          tunnel: [w1100] -> w1092
          tunnel: [w1099] -> w1091
          tunnel: w1090 -> [w1098]
          i -> [w1097]
          n569 = property on="产品参数列表（点击表格内任意位置，即可选中所对应产品）" class="Tbl (严格)"() -> ("Column Headers[]"=w1107:string[], "Value"=w1103:string[][])  [unwired: 2 in, 2 out]
          n570 = Index Array(array=w1107, index=w1098) -> (element=w1106:string)
          n571 = Number To Decimal String(number=w1097) -> (decimal integer string=w1105:string)  [unwired: 1 in]
          n572 = Decrement(x=w1097) -> (x-1=w1096:i32)
          n573 = Concatenate Strings(w1106, w1105) -> (w1104:string)
          n574 = call-poly <vilib>:"Read Key.vi"("section"="Setup", "error in (no error)"=w1109, "key"=w1104, "refnum"=w1110) -> ("error out"=w1099:errorcluster, "value"=w1101:string, "refnum out"=w1100:T4)  [unwired: 4 in, 1 out]
          n575 = Replace Array Subset(array=w1103, new element=w1101, index (row)=w1096, index (col)=w1098) -> (w1102:string[][])
          n576 = property on="产品参数列表（点击表格内任意位置，即可选中所对应产品）" class="Tbl (严格)"("Value"=w1102) -> ()  [unwired: 2 in, 2 out]
        }
      }
      n577 = for {
        N: w1067 -> [_]
        shift-right: [w1155] -> _
        shift-left: 0.0 -> [w1156]
        shift-right: [w1152] -> w1064
        shift-left: w1065 -> [w1153]
        i -> [w1157]
        n578 = Increment(x=w1156) -> (x+1=w1155:dbl)
        n579 = Number To Decimal String(number=w1155, width (-)=i16 3 ("宽度(-)")) -> (decimal integer string=w1154:string)
        n580 = Replace Array Subset(array=w1153, new element=w1154, index=w1157) -> (w1152:string[])
      }
      n581 = Build Array("日期", "序号", "二维码", "扭矩1", "角度1", "扭矩2", "角度2", "扭矩3", "角度3", "扭矩4", "角度4", "扭矩5", "角度5", "扭矩6", "角度6", "扭矩7", "角度7", "结果", "产品型号", "人员") -> (w1021:string[])
      n582 = Build Array("产品型号", "二维码规则", "二维码长度", "最小扭矩(N.m)", "最大扭矩(N.m)", "最小角度(°）", "最大角度(°）", "螺栓数量", "机器人程序号") -> (w1013:string[])
      n583 = property on="作业员列表" class="Tbl (严格)"("Row Headers[]"=w1053, "Column Headers[]"=string[] ["作业员编码", "作业员姓名", "", "", "", "", "", "", "", ""] ("列首字符串[]")) -> ()  [unwired: 2 in, 2 out]
      n584 = property on="产品参数列表（点击表格内任意位置，即可选中所对应产品）" class="Tbl (严格)"("Row Headers[]"=w1051, "Column Headers[]"=w1013) -> ()  [unwired: 2 in, 2 out]
      n585 = property on="表格" class="Tbl (严格)"("Row Headers[]"=w1064, "Column Headers[]"=w1021) -> ()  [unwired: 2 in, 2 out]
      n586 = property on="已选产品" class="Tbl (严格)"("Row Headers[]"=w1051, "Column Headers[]"=w1013, "Height"=u32 35 ("大小:高度")) -> ()  [unwired: 2 in, 2 out]
      n587 = call <vilib>:"Close Config Data.vi"("error in (no error)"=w1001, "refnum"=w1002) -> ()  [unwired: 8 in, 2 out]
      n588 = call <vilib>:"Close Config Data.vi"("error in (no error)"=w998, "refnum"=w997) -> ()  [unwired: 8 in, 2 out]
      "扭矩3合格" <- w984
      "扭矩1合格" <- w984
      "扭矩2合格" <- w984
      "扭矩4合格" <- w984
      "二维码" <- ""
      "字符串" <- "奥特佳新能源科技股份有限公司" ("字符串")
      "扭矩5合格" <- w984
      "扭矩6合格" <- w984
      "扭矩7合格" <- w984
    }
    frame #4 {
      n589 = while {
        stop <- FALSE stop-if-true
        n590 = event shown="[1] \"作业员 Operator\": 值改变" {
          selector: _ -> [_ _]
          dyn-events: _ -> [_ _]
          timeout: _ -> [_ _]
          event Timeout {
            n591 = event-data() -> ()  [unwired: 1 in, 3 out]
          }
          event "作业员 Operator": Value Change {
            n592 = event-data() -> ()  [unwired: 1 in, 6 out]
            n593 = Initialize Array("", 10 ("维数大小")) -> (w1204:string[])
            n594 = for {
              N: 10 -> [_]
              shift-right: [w1205] -> _
              shift-left: w1204 -> [w1208]
              i -> [w1207]
              n595 = local read "作业员列表"() -> (w1209:string[][])
              n596 = Index Array(array=w1209, index (row)=w1207, index (col)=1 ("禁用的索引 (列)")) -> (element=w1206:string)
              n597 = Replace Array Subset(array=w1208, new element=w1206, index=w1207) -> (w1205:string[])
              n598 = property on="作业员 Operator" class="Ring (严格)"("Strings []"=w1205) -> ()  [unwired: 2 in, 2 out]
            }
          }
        }
        n599 = Wait (ms)(milliseconds to wait=u32 250 ("等待时间（毫秒）")) -> ()  [unwired: 1 out]
      }
      n600 = while {
        stop <- FALSE stop-if-true
        n601 = Wait (ms)(milliseconds to wait=u32 1000 ("等待时间（毫秒）")) -> ()  [unwired: 1 out]
        n602 = for {
          N: 1000 -> [_]
          i -> [w1222]
          n603 = local read "表格"() -> (w1227:string[][])
          n604 = Wait (ms)(milliseconds to wait=u32 100 ("等待时间（毫秒）")) -> ()  [unwired: 1 out]
          n605 = Index Array(array=w1227, index (row)=w1222, index (col)=18 ("禁用的索引 (列)")) -> (element=w1216:string)
          n606 = Search and Replace String(input string=w1216, search string="OK" ("搜索字符串")) -> (number of replacements=w1224:i32)  [unwired: 6 in, 3 out]
          n607 = Search and Replace String(input string=w1216, search string="NG" ("搜索字符串")) -> (number of replacements=w1218:i32)  [unwired: 6 in, 3 out]
          n608 = Equal?(x=w1224, y=1) -> (x = y?=w1221:bool)
          n609 = Equal?(x=w1218, y=1) -> (x = y?=w1215:bool)
          n610 = case shown="False" w1221 {
            tunnel: w1222 -> [w1230 w1249]
            tunnel: "活动单元格:活动单元格" -> [w1229 w1247]
            tunnel: w1215 -> [w1228 _]
            frame False {
              n611 = case shown="False" w1228 {
                tunnel: w1230 -> [w1231 w1240]
                tunnel: w1229 -> [w1232 w1239]
                frame False {
                  n612 = for {
                    N: 10 -> [_]
                    tunnel: w1231 -> [w1238]
                    tunnel: w1232 -> [w1236]
                    i -> [w1237]
                    n613 = Bundle(cluster=w1236, "Row"=w1238, "Column"=w1237) -> (w1235:T2)
                    n614 = property on="表格" class="Tbl (严格)"("Active Cell"=w1235, "Cell BG Color"=u32 16777225 ("活动单元格:单元格背景色")) -> ()  [unwired: 2 in, 2 out]
                  }
                }
                frame True {
                  n615 = for {
                    N: 10 -> [_]
                    tunnel: w1240 -> [w1246]
                    tunnel: w1239 -> [w1244]
                    i -> [w1245]
                    n616 = Bundle(cluster=w1244, "Row"=w1246, "Column"=w1245) -> (w1243:T2)
                    n617 = property on="表格" class="Tbl (严格)"("Active Cell"=w1243, "Cell BG Color"=u32 16711680 ("活动单元格:单元格背景色")) -> ()  [unwired: 2 in, 2 out]
                  }
                }
              }
            }
            frame True {
              n618 = for {
                N: 10 -> [_]
                tunnel: w1249 -> [w1254]
                tunnel: w1247 -> [w1252]
                i -> [w1253]
                n619 = Bundle(cluster=w1252, "Row"=w1254, "Column"=w1253) -> (w1251:T2)
                n620 = property on="表格" class="Tbl (严格)"("Active Cell"=w1251, "Cell BG Color"=u32 6618880 ("活动单元格:单元格背景色")) -> ()  [unwired: 2 in, 2 out]
              }
            }
          }
        }
      }
      n621 = while {
        stop <- FALSE stop-if-true
        n622 = event shown="[1] \"产品参数列表（点击表格内任意位置，即可选中所对应产品）\": 鼠标按下" {
          selector: _ -> [_ _]
          dyn-events: _ -> [_ _]
          timeout: _ -> [_ _]
          event Timeout {
            n623 = event-data() -> ()  [unwired: 1 in, 3 out]
          }
          event "产品参数列表（点击表格内任意位置，即可选中所对应产品）": Mouse Down {
            n624 = event-data() -> ("Coords"=w1191:T13)  [unwired: 1 in, 7 out]
            n625 = invoke on="产品参数列表（点击表格内任意位置，即可选中所对应产品）" class="Tbl (严格)" method="Point To Row Column"("Point"=w1191) -> ("CellPosition"=w1190:T2)  [unwired: 5 in, 5 out]
            n626 = local read "产品参数列表（点击表格内任意位置，即可选中所对应产品）"() -> (w1188:string[][])
            n627 = Unbundle By Name(w1190) -> ("Row"=w1178:i32)
            n628 = Increment(x=w1178) -> (x+1=w1182:i32)
            "产品型号选择" <- w1182
            n629 = for {
              N: 9 -> [_]
              shift-right: [w1193] -> _
              shift-left: "已选产品" -> [w1194]
              tunnel: w1188 -> [w1197]
              tunnel: w1178 -> [w1196]
              tunnel: [w1193] -> w1176
              i -> [w1192]
              n630 = Index Array(array=w1197, index (row)=w1196, index (col)=w1192) -> (element=w1195:string)
              n631 = Replace Array Subset(array=w1194, new element=w1195, index (row)=0 ("禁用的索引 (行)"), index (col)=w1192) -> (w1193:string[][])
            }
            n632 = Number To Decimal String(number=w1182) -> (decimal integer string=w1179:string)  [unwired: 1 in]
            n633 = Index Array(array=w1176, index (row)=0 ("索引 (行)"), index (col)=7 ("索引 (行)")) -> (element=w1184:string)
            n634 = Decimal String To Number(string=w1184) -> (number=→"螺栓数量":i32)  [unwired: 2 in, 1 out]
            n635 = Replace Array Subset(array=w1176, new element=w1179, index (row)=0 ("禁用的索引 (行)"), index (col)=8 ("禁用的索引 (列)")) -> (w1181:string[][])
            n636 = local write "已选产品"(w1181) -> ()
          }
        }
        n637 = Wait (ms)(milliseconds to wait=u32 250 ("等待时间（毫秒）")) -> ()  [unwired: 1 out]
      }
      n638 = local read "产品参数列表（点击表格内任意位置，即可选中所对应产品）"() -> (w1162:string[][])
      n639 = local read "已选产品"() -> (w1158:string[][])
      n640 = for {
        N: 8 -> [_]
        shift-right: [w1167] -> _
        shift-left: w1158 -> [w1168]
        tunnel: w1162 -> [w1172]
        tunnel: 0 ("Row") -> [w1171]
        tunnel: [w1167] -> w1163
        i -> [w1170]
        n641 = Index Array(array=w1172, index (row)=w1171, index (col)=w1170) -> (element=w1169:string)
        n642 = Replace Array Subset(array=w1168, new element=w1169, index (row)=0 ("禁用的索引 (行)"), index (col)=w1170) -> (w1167:string[][])
        n643 = local write "已选产品"(w1167) -> ()
      }
      n644 = Index Array(array=w1163, index (row)=0 ("索引 (行)"), index (col)=7 ("索引 (行)")) -> (element=w1166:string)
      n645 = Decimal String To Number(string=w1166) -> (number=w1159:i32)  [unwired: 2 in, 1 out]
      n646 = shared-variable "我的电脑\\opc.lvlib\\螺栓数量"(w1159) -> ()  [unwired: 1 in, 1 out]
    }
  }
  n647 = while {
    stop <- FALSE stop-if-true
    n648 = local read "螺栓6扭矩读取"() -> (w1255:bool)
    n649 = local read "螺栓0扭矩读取"() -> (w1264:bool)
    n650 = local read "螺栓1扭矩读取"() -> (w1263:bool)
    n651 = local read "螺栓2扭矩读取"() -> (w1262:bool)
    n652 = local read "螺栓3扭矩读取"() -> (w1261:bool)
    n653 = local read "螺栓4扭矩读取"() -> (w1260:bool)
    n654 = local read "螺栓5扭矩读取"() -> (w1259:bool)
    n655 = Wait (ms)(milliseconds to wait=u32 10 ("等待时间（毫秒）")) -> ()  [unwired: 1 out]
    n656 = Compound Arithmetic op=OR ("复合运算")(w1264, w1263, w1262, w1261, w1260, w1259, w1255) -> (w1258:bool)
    n657 = case shown="1" "扭矩保存过程" {
      tunnel: w1258 -> [w1266 w1268 _]
      frame 0, Default {
        n658 = case shown="False" w1266 {
          frame False {
          }
          frame True {
            n659 = local write "扭矩保存过程"(u8 1 ("扭矩保存过程")) -> ()
          }
        }
      }
      frame 2 {
        n660 = case shown="False" w1268 {
          frame False {
            n661 = local write "扭矩保存过程"(u8 0 ("扭矩保存过程")) -> ()
          }
          frame True {
          }
        }
      }
      frame 1 {
        n662 = flat-sequence {
          tunnel: [w1629] -> w1270
          tunnel: [w1732] -> w1271
          tunnel: w1270 -> [w1732]
          tunnel: w1271 -> [w1734]
          frame #0 {
            n663 = local read "螺栓0扭矩读取"() -> (w1278:bool)
            n664 = local read "螺栓1扭矩读取"() -> (w1277:bool)
            n665 = local read "螺栓2扭矩读取"() -> (w1276:bool)
            n666 = local read "螺栓6扭矩读取"() -> (w1272:bool)
            n667 = local read "螺栓3扭矩读取"() -> (w1275:bool)
            n668 = local read "螺栓4扭矩读取"() -> (w1274:bool)
            n669 = local read "螺栓5扭矩读取"() -> (w1273:bool)
            n670 = case shown="True" w1278 {
              frame False {
              }
              frame True {
                n671 = for {
                  N: 2 -> [_]
                  tunnel: [w1549] -> w1532
                  tunnel: [w1547] -> w1530
                  tunnel: [w1546] -> w1529
                  w1571 = 0 ("禁用的索引 (列)")
                  n672 = local read "扭矩字符串"() -> (w1570:string)
                  n673 = local read "角度字符串"() -> (w1569:string)
                  n674 = local read "扭矩/角度"() -> (w1575:string[][])
                  n675 = local read "已选产品"() -> (w1560:string[][])
                  n676 = Wait (ms)(milliseconds to wait=u32 1000 ("等待时间（毫秒）")) -> ()  [unwired: 1 out]
                  n677 = Fract/Exp String To Number(string=w1570) -> (number=w1555:dbl)  [unwired: 3 in, 1 out]
                  n678 = Fract/Exp String To Number(string=w1569) -> (number=w1550:dbl)  [unwired: 3 in, 1 out]
                  n679 = Index Array(array=w1560, index (row)=0 ("索引 (行)"), index (col)=4 ("禁用的索引 (列)")) -> (element=w1558:string)
                  n680 = Index Array(array=w1560, index (row)=0 ("索引 (行)"), index (col)=3 ("禁用的索引 (列)")) -> (element=w1559:string)
                  n681 = Index Array(array=w1560, index (row)=0 ("索引 (行)"), index (col)=6 ("禁用的索引 (列)")) -> (element=w1554:string)
                  n682 = Index Array(array=w1560, index (row)=0 ("索引 (行)"), index (col)=5 ("禁用的索引 (列)")) -> (element=w1553:string)
                  n683 = Fract/Exp String To Number(string=w1558) -> (number=w1557:dbl)  [unwired: 3 in, 1 out]
                  n684 = Fract/Exp String To Number(string=w1559) -> (number=w1556:dbl)  [unwired: 3 in, 1 out]
                  n685 = Fract/Exp String To Number(string=w1554) -> (number=w1552:dbl)  [unwired: 3 in, 1 out]
                  n686 = Fract/Exp String To Number(string=w1553) -> (number=w1551:dbl)  [unwired: 3 in, 1 out]
                  n687 = Replace Array Subset(array=w1575, new element #1=w1570, index (row) #1=w1571, index (col) #1=0 ("禁用的索引 (列)"), new element #2=w1569, index (row) #2=w1571, index (col) #2=1 ("索引 (列)")) -> (w1574:string[][])
                  n688 = In Range and Coerce(upper limit=w1557, x=w1555, lower limit=w1556) -> (In Range?=w1547:bool)  [unwired: 1 out]
                  n689 = In Range and Coerce(upper limit=w1552, x=w1550, lower limit=w1551) -> (In Range?=w1546:bool)  [unwired: 1 out]
                  n690 = local write "扭矩/角度"(w1574) -> ()
                  n691 = And(x=w1547, y=w1546) -> (x .and. y?=w1549:bool)
                }
                n692 = Not(x=w1532) -> (.not. x?=→"螺栓0读取错误":bool)
                n693 = case shown="True" w1532 {
                  tunnel: w1532 -> [_ w1578]
                  frame False {
                    n694 = property on="扭矩1合格" class="Bool (严格)"("Colors [4]"=cluster{u32, u32}[] [{16711680, 16711680}] ("颜色[4]")) -> ()  [unwired: 2 in, 2 out]
                  }
                  frame True {
                    n695 = local write "扭矩1合格"(w1578) -> ()
                    n696 = property on="扭矩1合格" class="Bool (严格)"("Colors [4]"=cluster{u32, u32}[] [{6618880, 6618880}] ("颜色[4]")) -> ()  [unwired: 2 in, 2 out]
                  }
                }
                n697 = case shown="True" w1530 {
                  frame True {
                    n698 = local read "扭矩/角度"() -> (w1540:string[][])
                    n699 = property on="扭矩角度表格" class="Tbl (严格)"("Active Cell"=T2 {"Row"=0, "Column"=0} ("活动单元格:活动单元格"), "Cell BG Color"=u32 6618880 ("活动单元格:单元格背景色"), "Value"=w1540) -> ()  [unwired: 2 in, 2 out]
                  }
                  frame False {
                    n700 = local read "扭矩/角度"() -> (w1543:string[][])
                    n701 = property on="扭矩角度表格" class="Tbl (严格)"("Active Cell"=T2 {"Row"=0, "Column"=0} ("活动单元格:活动单元格"), "Cell BG Color"=u32 16711680 ("活动单元格:单元格背景色"), "Value"=w1543) -> ()  [unwired: 2 in, 2 out]
                  }
                }
                n702 = case shown="True" w1529 {
                  frame True {
                    n703 = local read "扭矩/角度"() -> (w1534:string[][])
                    n704 = property on="扭矩角度表格" class="Tbl (严格)"("Active Cell"=T2 {"Row"=0, "Column"=1} ("活动单元格:活动单元格"), "Cell BG Color"=u32 6618880 ("活动单元格:单元格背景色"), "Value"=w1534) -> ()  [unwired: 2 in, 2 out]
                  }
                  frame False {
                    n705 = local read "扭矩/角度"() -> (w1537:string[][])
                    n706 = property on="扭矩角度表格" class="Tbl (严格)"("Active Cell"=T2 {"Row"=0, "Column"=1} ("活动单元格:活动单元格"), "Cell BG Color"=u32 16711680 ("活动单元格:单元格背景色"), "Value"=w1537) -> ()  [unwired: 2 in, 2 out]
                  }
                }
              }
            }
            n707 = case shown="True" w1277 {
              frame False {
              }
              frame True {
                n708 = for {
                  N: 2 -> [_]
                  tunnel: [w1449] -> w1432
                  tunnel: [w1447] -> w1430
                  tunnel: [w1446] -> w1429
                  w1471 = 1 ("禁用的索引 (列)")
                  n709 = local read "扭矩字符串"() -> (w1470:string)
                  n710 = local read "角度字符串"() -> (w1469:string)
                  n711 = local read "扭矩/角度"() -> (w1475:string[][])
                  n712 = local read "已选产品"() -> (w1460:string[][])
                  n713 = Wait (ms)(milliseconds to wait=u32 1000 ("等待时间（毫秒）")) -> ()  [unwired: 1 out]
                  n714 = Fract/Exp String To Number(string=w1470) -> (number=w1455:dbl)  [unwired: 3 in, 1 out]
                  n715 = Fract/Exp String To Number(string=w1469) -> (number=w1450:dbl)  [unwired: 3 in, 1 out]
                  n716 = Index Array(array=w1460, index (row)=0 ("索引 (行)"), index (col)=4 ("禁用的索引 (列)")) -> (element=w1458:string)
                  n717 = Index Array(array=w1460, index (row)=0 ("索引 (行)"), index (col)=3 ("禁用的索引 (列)")) -> (element=w1459:string)
                  n718 = Index Array(array=w1460, index (row)=0 ("索引 (行)"), index (col)=6 ("禁用的索引 (列)")) -> (element=w1454:string)
                  n719 = Index Array(array=w1460, index (row)=0 ("索引 (行)"), index (col)=5 ("禁用的索引 (列)")) -> (element=w1453:string)
                  n720 = Fract/Exp String To Number(string=w1458) -> (number=w1457:dbl)  [unwired: 3 in, 1 out]
                  n721 = Fract/Exp String To Number(string=w1459) -> (number=w1456:dbl)  [unwired: 3 in, 1 out]
                  n722 = Fract/Exp String To Number(string=w1454) -> (number=w1452:dbl)  [unwired: 3 in, 1 out]
                  n723 = Fract/Exp String To Number(string=w1453) -> (number=w1451:dbl)  [unwired: 3 in, 1 out]
                  n724 = Replace Array Subset(array=w1475, new element #1=w1470, index (row) #1=w1471, index (col) #1=0 ("禁用的索引 (列)"), new element #2=w1469, index (row) #2=w1471, index (col) #2=1 ("索引 (列)")) -> (w1474:string[][])
                  n725 = In Range and Coerce(upper limit=w1457, x=w1455, lower limit=w1456) -> (In Range?=w1447:bool)  [unwired: 1 out]
                  n726 = In Range and Coerce(upper limit=w1452, x=w1450, lower limit=w1451) -> (In Range?=w1446:bool)  [unwired: 1 out]
                  n727 = local write "扭矩/角度"(w1474) -> ()
                  n728 = And(x=w1447, y=w1446) -> (x .and. y?=w1449:bool)
                }
                n729 = Not(x=w1432) -> (.not. x?=→"螺栓1读取错误":bool)
                n730 = case shown="False" w1432 {
                  tunnel: w1432 -> [_ w1478]
                  frame False {
                    n731 = property on="扭矩2合格" class="Bool (严格)"("Colors [4]"=cluster{u32, u32}[] [{16711680, 16711680}] ("颜色[4]")) -> ()  [unwired: 2 in, 2 out]
                  }
                  frame True {
                    n732 = local write "扭矩2合格"(w1478) -> ()
                    n733 = property on="扭矩2合格" class="Bool (严格)"("Colors [4]"=cluster{u32, u32}[] [{6618880, 6618880}] ("颜色[4]")) -> ()  [unwired: 2 in, 2 out]
                  }
                }
                n734 = case shown="True" w1430 {
                  frame True {
                    n735 = local read "扭矩/角度"() -> (w1440:string[][])
                    n736 = property on="扭矩角度表格" class="Tbl (严格)"("Active Cell"=T2 {"Row"=1, "Column"=0} ("活动单元格:活动单元格"), "Cell BG Color"=u32 6618880 ("活动单元格:单元格背景色"), "Value"=w1440) -> ()  [unwired: 2 in, 2 out]
                  }
                  frame False {
                    n737 = local read "扭矩/角度"() -> (w1443:string[][])
                    n738 = property on="扭矩角度表格" class="Tbl (严格)"("Active Cell"=T2 {"Row"=1, "Column"=0} ("活动单元格:活动单元格"), "Cell BG Color"=u32 16711680 ("活动单元格:单元格背景色"), "Value"=w1443) -> ()  [unwired: 2 in, 2 out]
                  }
                }
                n739 = case shown="True" w1429 {
                  frame True {
                    n740 = local read "扭矩/角度"() -> (w1434:string[][])
                    n741 = property on="扭矩角度表格" class="Tbl (严格)"("Active Cell"=T2 {"Row"=1, "Column"=1} ("活动单元格:活动单元格"), "Cell BG Color"=u32 6618880 ("活动单元格:单元格背景色"), "Value"=w1434) -> ()  [unwired: 2 in, 2 out]
                  }
                  frame False {
                    n742 = local read "扭矩/角度"() -> (w1437:string[][])
                    n743 = property on="扭矩角度表格" class="Tbl (严格)"("Active Cell"=T2 {"Row"=1, "Column"=1} ("活动单元格:活动单元格"), "Cell BG Color"=u32 16711680 ("活动单元格:单元格背景色"), "Value"=w1437) -> ()  [unwired: 2 in, 2 out]
                  }
                }
              }
            }
            n744 = case shown="True" w1276 {
              frame False {
              }
              frame True {
                n745 = for {
                  N: 2 -> [_]
                  tunnel: [w1349] -> w1332
                  tunnel: [w1347] -> w1330
                  tunnel: [w1346] -> w1329
                  w1371 = 2 ("禁用的索引 (列)")
                  n746 = local read "扭矩字符串"() -> (w1370:string)
                  n747 = local read "角度字符串"() -> (w1369:string)
                  n748 = local read "扭矩/角度"() -> (w1375:string[][])
                  n749 = local read "已选产品"() -> (w1360:string[][])
                  n750 = Wait (ms)(milliseconds to wait=u32 1000 ("等待时间（毫秒）")) -> ()  [unwired: 1 out]
                  n751 = Fract/Exp String To Number(string=w1370) -> (number=w1355:dbl)  [unwired: 3 in, 1 out]
                  n752 = Fract/Exp String To Number(string=w1369) -> (number=w1350:dbl)  [unwired: 3 in, 1 out]
                  n753 = Index Array(array=w1360, index (row)=0 ("索引 (行)"), index (col)=4 ("禁用的索引 (列)")) -> (element=w1358:string)
                  n754 = Index Array(array=w1360, index (row)=0 ("索引 (行)"), index (col)=3 ("禁用的索引 (列)")) -> (element=w1359:string)
                  n755 = Index Array(array=w1360, index (row)=0 ("索引 (行)"), index (col)=6 ("禁用的索引 (列)")) -> (element=w1354:string)
                  n756 = Index Array(array=w1360, index (row)=0 ("索引 (行)"), index (col)=5 ("禁用的索引 (列)")) -> (element=w1353:string)
                  n757 = Fract/Exp String To Number(string=w1358) -> (number=w1357:dbl)  [unwired: 3 in, 1 out]
                  n758 = Fract/Exp String To Number(string=w1359) -> (number=w1356:dbl)  [unwired: 3 in, 1 out]
                  n759 = Fract/Exp String To Number(string=w1354) -> (number=w1352:dbl)  [unwired: 3 in, 1 out]
                  n760 = Fract/Exp String To Number(string=w1353) -> (number=w1351:dbl)  [unwired: 3 in, 1 out]
                  n761 = Replace Array Subset(array=w1375, new element #1=w1370, index (row) #1=w1371, index (col) #1=0 ("禁用的索引 (列)"), new element #2=w1369, index (row) #2=w1371, index (col) #2=1 ("索引 (列)")) -> (w1374:string[][])
                  n762 = In Range and Coerce(upper limit=w1357, x=w1355, lower limit=w1356) -> (In Range?=w1346:bool)  [unwired: 1 out]
                  n763 = In Range and Coerce(upper limit=w1352, x=w1350, lower limit=w1351) -> (In Range?=w1347:bool)  [unwired: 1 out]
                  n764 = local write "扭矩/角度"(w1374) -> ()
                  n765 = And(x=w1346, y=w1347) -> (x .and. y?=w1349:bool)
                }
                n766 = Not(x=w1332) -> (.not. x?=→"螺栓2读取错误":bool)
                n767 = case shown="False" w1332 {
                  tunnel: w1332 -> [_ w1378]
                  frame False {
                    n768 = property on="扭矩3合格" class="Bool (严格)"("Colors [4]"=cluster{u32, u32}[] [{16711680, 16711680}] ("颜色[4]")) -> ()  [unwired: 2 in, 2 out]
                  }
                  frame True {
                    n769 = local write "扭矩3合格"(w1378) -> ()
                    n770 = property on="扭矩3合格" class="Bool (严格)"("Colors [4]"=cluster{u32, u32}[] [{6618880, 6618880}] ("颜色[4]")) -> ()  [unwired: 2 in, 2 out]
                  }
                }
                n771 = case shown="True" w1329 {
                  frame True {
                    n772 = local read "扭矩/角度"() -> (w1340:string[][])
                    n773 = property on="扭矩角度表格" class="Tbl (严格)"("Active Cell"=T2 {"Row"=2, "Column"=0} ("活动单元格:活动单元格"), "Cell BG Color"=u32 6618880 ("活动单元格:单元格背景色"), "Value"=w1340) -> ()  [unwired: 2 in, 2 out]
                  }
                  frame False {
                    n774 = local read "扭矩/角度"() -> (w1343:string[][])
                    n775 = property on="扭矩角度表格" class="Tbl (严格)"("Active Cell"=T2 {"Row"=2, "Column"=0} ("活动单元格:活动单元格"), "Cell BG Color"=u32 16711680 ("活动单元格:单元格背景色"), "Value"=w1343) -> ()  [unwired: 2 in, 2 out]
                  }
                }
                n776 = case shown="True" w1330 {
                  frame True {
                    n777 = local read "扭矩/角度"() -> (w1334:string[][])
                    n778 = property on="扭矩角度表格" class="Tbl (严格)"("Active Cell"=T2 {"Row"=2, "Column"=1} ("活动单元格:活动单元格"), "Cell BG Color"=u32 6618880 ("活动单元格:单元格背景色"), "Value"=w1334) -> ()  [unwired: 2 in, 2 out]
                  }
                  frame False {
                    n779 = local read "扭矩/角度"() -> (w1337:string[][])
                    n780 = property on="扭矩角度表格" class="Tbl (严格)"("Active Cell"=T2 {"Row"=2, "Column"=1} ("活动单元格:活动单元格"), "Cell BG Color"=u32 16711680 ("活动单元格:单元格背景色"), "Value"=w1337) -> ()  [unwired: 2 in, 2 out]
                  }
                }
              }
            }
            n781 = case shown="True" w1272 {
              frame False {
              }
              frame True {
                n782 = for {
                  N: 2 -> [_]
                  tunnel: [w1299] -> w1283
                  tunnel: [w1297] -> w1281
                  tunnel: [w1296] -> w1280
                  w1321 = 6 ("禁用的索引 (列)")
                  n783 = local read "扭矩字符串"() -> (w1320:string)
                  n784 = local read "角度字符串"() -> (w1319:string)
                  n785 = local read "扭矩/角度"() -> (w1325:string[][])
                  n786 = local read "已选产品"() -> (w1310:string[][])
                  n787 = Wait (ms)(milliseconds to wait=u32 1000 ("等待时间（毫秒）")) -> ()  [unwired: 1 out]
                  n788 = Fract/Exp String To Number(string=w1320) -> (number=w1305:dbl)  [unwired: 3 in, 1 out]
                  n789 = Fract/Exp String To Number(string=w1319) -> (number=w1300:dbl)  [unwired: 3 in, 1 out]
                  n790 = Index Array(array=w1310, index (row)=0 ("索引 (行)"), index (col)=4 ("禁用的索引 (列)")) -> (element=w1308:string)
                  n791 = Index Array(array=w1310, index (row)=0 ("索引 (行)"), index (col)=3 ("禁用的索引 (列)")) -> (element=w1309:string)
                  n792 = Index Array(array=w1310, index (row)=0 ("索引 (行)"), index (col)=6 ("禁用的索引 (列)")) -> (element=w1304:string)
                  n793 = Index Array(array=w1310, index (row)=0 ("索引 (行)"), index (col)=5 ("禁用的索引 (列)")) -> (element=w1303:string)
                  n794 = Fract/Exp String To Number(string=w1308) -> (number=w1307:dbl)  [unwired: 3 in, 1 out]
                  n795 = Fract/Exp String To Number(string=w1309) -> (number=w1306:dbl)  [unwired: 3 in, 1 out]
                  n796 = Fract/Exp String To Number(string=w1304) -> (number=w1302:dbl)  [unwired: 3 in, 1 out]
                  n797 = Fract/Exp String To Number(string=w1303) -> (number=w1301:dbl)  [unwired: 3 in, 1 out]
                  n798 = Replace Array Subset(array=w1325, new element #1=w1320, index (row) #1=w1321, index (col) #1=0 ("禁用的索引 (列)"), new element #2=w1319, index (row) #2=w1321, index (col) #2=1 ("索引 (列)")) -> (w1324:string[][])
                  n799 = In Range and Coerce(upper limit=w1307, x=w1305, lower limit=w1306) -> (In Range?=w1296:bool)  [unwired: 1 out]
                  n800 = In Range and Coerce(upper limit=w1302, x=w1300, lower limit=w1301) -> (In Range?=w1297:bool)  [unwired: 1 out]
                  n801 = local write "扭矩/角度"(w1324) -> ()
                  n802 = And(x=w1296, y=w1297) -> (x .and. y?=w1299:bool)
                }
                n803 = Not(x=w1283) -> (.not. x?=→"螺栓6读取错误":bool)
                n804 = case shown="True" w1283 {
                  tunnel: w1283 -> [_ w1328]
                  frame False {
                    n805 = property on="扭矩7合格" class="Bool (严格)"("Colors [4]"=cluster{u32, u32}[] [{16711680, 16711680}] ("颜色[4]")) -> ()  [unwired: 2 in, 2 out]
                  }
                  frame True {
                    n806 = local write "扭矩7合格"(w1328) -> ()
                    n807 = property on="扭矩7合格" class="Bool (严格)"("Colors [4]"=cluster{u32, u32}[] [{6618880, 6618880}] ("颜色[4]")) -> ()  [unwired: 2 in, 2 out]
                  }
                }
                n808 = case shown="True" w1280 {
                  frame True {
                    n809 = local read "扭矩/角度"() -> (w1290:string[][])
                    n810 = property on="扭矩角度表格" class="Tbl (严格)"("Active Cell"=T2 {"Row"=6, "Column"=0} ("活动单元格:活动单元格"), "Cell BG Color"=u32 6618880 ("活动单元格:单元格背景色"), "Value"=w1290) -> ()  [unwired: 2 in, 2 out]
                  }
                  frame False {
                    n811 = local read "扭矩/角度"() -> (w1293:string[][])
                    n812 = property on="扭矩角度表格" class="Tbl (严格)"("Active Cell"=T2 {"Row"=6, "Column"=0} ("活动单元格:活动单元格"), "Cell BG Color"=u32 16711680 ("活动单元格:单元格背景色"), "Value"=w1293) -> ()  [unwired: 2 in, 2 out]
                  }
                }
                n813 = case shown="True" w1281 {
                  frame True {
                    n814 = local read "扭矩/角度"() -> (w1284:string[][])
                    n815 = property on="扭矩角度表格" class="Tbl (严格)"("Active Cell"=T2 {"Row"=6, "Column"=1} ("活动单元格:活动单元格"), "Cell BG Color"=u32 6618880 ("活动单元格:单元格背景色"), "Value"=w1284) -> ()  [unwired: 2 in, 2 out]
                  }
                  frame False {
                    n816 = local read "扭矩/角度"() -> (w1287:string[][])
                    n817 = property on="扭矩角度表格" class="Tbl (严格)"("Active Cell"=T2 {"Row"=6, "Column"=1} ("活动单元格:活动单元格"), "Cell BG Color"=u32 16711680 ("活动单元格:单元格背景色"), "Value"=w1287) -> ()  [unwired: 2 in, 2 out]
                  }
                }
              }
            }
            n818 = case shown="True" w1275 {
              frame False {
              }
              frame True {
                n819 = for {
                  N: 2 -> [_]
                  tunnel: [w1599] -> w1582
                  tunnel: [w1597] -> w1580
                  tunnel: [w1596] -> w1579
                  w1621 = 3 ("禁用的索引 (列)")
                  n820 = local read "扭矩字符串"() -> (w1620:string)
                  n821 = local read "角度字符串"() -> (w1619:string)
                  n822 = local read "扭矩/角度"() -> (w1625:string[][])
                  n823 = local read "已选产品"() -> (w1610:string[][])
                  n824 = Wait (ms)(milliseconds to wait=u32 1000 ("等待时间（毫秒）")) -> ()  [unwired: 1 out]
                  n825 = Fract/Exp String To Number(string=w1620) -> (number=w1605:dbl)  [unwired: 3 in, 1 out]
                  n826 = Fract/Exp String To Number(string=w1619) -> (number=w1600:dbl)  [unwired: 3 in, 1 out]
                  n827 = Index Array(array=w1610, index (row)=0 ("索引 (行)"), index (col)=4 ("禁用的索引 (列)")) -> (element=w1608:string)
                  n828 = Index Array(array=w1610, index (row)=0 ("索引 (行)"), index (col)=3 ("禁用的索引 (列)")) -> (element=w1609:string)
                  n829 = Index Array(array=w1610, index (row)=0 ("索引 (行)"), index (col)=6 ("禁用的索引 (列)")) -> (element=w1604:string)
                  n830 = Index Array(array=w1610, index (row)=0 ("索引 (行)"), index (col)=5 ("禁用的索引 (列)")) -> (element=w1603:string)
                  n831 = Fract/Exp String To Number(string=w1608) -> (number=w1607:dbl)  [unwired: 3 in, 1 out]
                  n832 = Fract/Exp String To Number(string=w1609) -> (number=w1606:dbl)  [unwired: 3 in, 1 out]
                  n833 = Fract/Exp String To Number(string=w1604) -> (number=w1602:dbl)  [unwired: 3 in, 1 out]
                  n834 = Fract/Exp String To Number(string=w1603) -> (number=w1601:dbl)  [unwired: 3 in, 1 out]
                  n835 = Replace Array Subset(array=w1625, new element #1=w1620, index (row) #1=w1621, index (col) #1=0 ("禁用的索引 (列)"), new element #2=w1619, index (row) #2=w1621, index (col) #2=1 ("索引 (列)")) -> (w1624:string[][])
                  n836 = In Range and Coerce(upper limit=w1607, x=w1605, lower limit=w1606) -> (In Range?=w1596:bool)  [unwired: 1 out]
                  n837 = In Range and Coerce(upper limit=w1602, x=w1600, lower limit=w1601) -> (In Range?=w1597:bool)  [unwired: 1 out]
                  n838 = local write "扭矩/角度"(w1624) -> ()
                  n839 = And(x=w1596, y=w1597) -> (x .and. y?=w1599:bool)
                }
                n840 = Not(x=w1582) -> (.not. x?=→"螺栓3读取错误":bool)
                n841 = case shown="False" w1582 {
                  tunnel: w1582 -> [_ w1628]
                  frame False {
                    n842 = property on="扭矩4合格" class="Bool (严格)"("Colors [4]"=cluster{u32, u32}[] [{16711680, 16711680}] ("颜色[4]")) -> ()  [unwired: 2 in, 2 out]
                  }
                  frame True {
                    n843 = local write "扭矩4合格"(w1628) -> ()
                    n844 = property on="扭矩4合格" class="Bool (严格)"("Colors [4]"=cluster{u32, u32}[] [{6618880, 6618880}] ("颜色[4]")) -> ()  [unwired: 2 in, 2 out]
                  }
                }
                n845 = case shown="False" w1579 {
                  frame True {
                    n846 = local read "扭矩/角度"() -> (w1590:string[][])
                    n847 = property on="扭矩角度表格" class="Tbl (严格)"("Active Cell"=T2 {"Row"=3, "Column"=0} ("活动单元格:活动单元格"), "Cell BG Color"=u32 6618880 ("活动单元格:单元格背景色"), "Value"=w1590) -> ()  [unwired: 2 in, 2 out]
                  }
                  frame False {
                    n848 = local read "扭矩/角度"() -> (w1593:string[][])
                    n849 = property on="扭矩角度表格" class="Tbl (严格)"("Active Cell"=T2 {"Row"=3, "Column"=0} ("活动单元格:活动单元格"), "Cell BG Color"=u32 16711680 ("活动单元格:单元格背景色"), "Value"=w1593) -> ()  [unwired: 2 in, 2 out]
                  }
                }
                n850 = case shown="False" w1580 {
                  frame True {
                    n851 = local read "扭矩/角度"() -> (w1584:string[][])
                    n852 = property on="扭矩角度表格" class="Tbl (严格)"("Active Cell"=T2 {"Row"=3, "Column"=1} ("活动单元格:活动单元格"), "Cell BG Color"=u32 6618880 ("活动单元格:单元格背景色"), "Value"=w1584) -> ()  [unwired: 2 in, 2 out]
                  }
                  frame False {
                    n853 = local read "扭矩/角度"() -> (w1587:string[][])
                    n854 = property on="扭矩角度表格" class="Tbl (严格)"("Active Cell"=T2 {"Row"=3, "Column"=1} ("活动单元格:活动单元格"), "Cell BG Color"=u32 16711680 ("活动单元格:单元格背景色"), "Value"=w1587) -> ()  [unwired: 2 in, 2 out]
                  }
                }
              }
            }
            n855 = case shown="True" w1274 {
              frame False {
              }
              frame True {
                n856 = for {
                  N: 2 -> [_]
                  tunnel: [w1499] -> w1482
                  tunnel: [w1497] -> w1480
                  tunnel: [w1496] -> w1479
                  w1521 = 4 ("禁用的索引 (列)")
                  n857 = local read "扭矩字符串"() -> (w1520:string)
                  n858 = local read "角度字符串"() -> (w1519:string)
                  n859 = local read "扭矩/角度"() -> (w1525:string[][])
                  n860 = local read "已选产品"() -> (w1510:string[][])
                  n861 = Wait (ms)(milliseconds to wait=u32 1000 ("等待时间（毫秒）")) -> ()  [unwired: 1 out]
                  n862 = Fract/Exp String To Number(string=w1520) -> (number=w1505:dbl)  [unwired: 3 in, 1 out]
                  n863 = Fract/Exp String To Number(string=w1519) -> (number=w1500:dbl)  [unwired: 3 in, 1 out]
                  n864 = Index Array(array=w1510, index (row)=0 ("索引 (行)"), index (col)=4 ("禁用的索引 (列)")) -> (element=w1508:string)
                  n865 = Index Array(array=w1510, index (row)=0 ("索引 (行)"), index (col)=3 ("禁用的索引 (列)")) -> (element=w1509:string)
                  n866 = Index Array(array=w1510, index (row)=0 ("索引 (行)"), index (col)=6 ("禁用的索引 (列)")) -> (element=w1504:string)
                  n867 = Index Array(array=w1510, index (row)=0 ("索引 (行)"), index (col)=5 ("禁用的索引 (列)")) -> (element=w1503:string)
                  n868 = Fract/Exp String To Number(string=w1508) -> (number=w1507:dbl)  [unwired: 3 in, 1 out]
                  n869 = Fract/Exp String To Number(string=w1509) -> (number=w1506:dbl)  [unwired: 3 in, 1 out]
                  n870 = Fract/Exp String To Number(string=w1504) -> (number=w1502:dbl)  [unwired: 3 in, 1 out]
                  n871 = Fract/Exp String To Number(string=w1503) -> (number=w1501:dbl)  [unwired: 3 in, 1 out]
                  n872 = Replace Array Subset(array=w1525, new element #1=w1520, index (row) #1=w1521, index (col) #1=0 ("禁用的索引 (列)"), new element #2=w1519, index (row) #2=w1521, index (col) #2=1 ("索引 (列)")) -> (w1524:string[][])
                  n873 = In Range and Coerce(upper limit=w1507, x=w1505, lower limit=w1506) -> (In Range?=w1496:bool)  [unwired: 1 out]
                  n874 = In Range and Coerce(upper limit=w1502, x=w1500, lower limit=w1501) -> (In Range?=w1497:bool)  [unwired: 1 out]
                  n875 = local write "扭矩/角度"(w1524) -> ()
                  n876 = And(x=w1496, y=w1497) -> (x .and. y?=w1499:bool)
                }
                n877 = Not(x=w1482) -> (.not. x?=→"螺栓4读取错误":bool)
                n878 = case shown="False" w1482 {
                  tunnel: w1482 -> [_ w1528]
                  frame False {
                    n879 = property on="扭矩5合格" class="Bool (严格)"("Colors [4]"=cluster{u32, u32}[] [{16711680, 16711680}] ("颜色[4]")) -> ()  [unwired: 2 in, 2 out]
                  }
                  frame True {
                    n880 = local write "扭矩5合格"(w1528) -> ()
                    n881 = property on="扭矩5合格" class="Bool (严格)"("Colors [4]"=cluster{u32, u32}[] [{6618880, 6618880}] ("颜色[4]")) -> ()  [unwired: 2 in, 2 out]
                  }
                }
                n882 = case shown="True" w1479 {
                  frame True {
                    n883 = local read "扭矩/角度"() -> (w1490:string[][])
                    n884 = property on="扭矩角度表格" class="Tbl (严格)"("Active Cell"=T2 {"Row"=4, "Column"=0} ("活动单元格:活动单元格"), "Cell BG Color"=u32 6618880 ("活动单元格:单元格背景色"), "Value"=w1490) -> ()  [unwired: 2 in, 2 out]
                  }
                  frame False {
                    n885 = local read "扭矩/角度"() -> (w1493:string[][])
                    n886 = property on="扭矩角度表格" class="Tbl (严格)"("Active Cell"=T2 {"Row"=4, "Column"=0} ("活动单元格:活动单元格"), "Cell BG Color"=u32 16711680 ("活动单元格:单元格背景色"), "Value"=w1493) -> ()  [unwired: 2 in, 2 out]
                  }
                }
                n887 = case shown="True" w1480 {
                  frame True {
                    n888 = local read "扭矩/角度"() -> (w1484:string[][])
                    n889 = property on="扭矩角度表格" class="Tbl (严格)"("Active Cell"=T2 {"Row"=4, "Column"=1} ("活动单元格:活动单元格"), "Cell BG Color"=u32 6618880 ("活动单元格:单元格背景色"), "Value"=w1484) -> ()  [unwired: 2 in, 2 out]
                  }
                  frame False {
                    n890 = local read "扭矩/角度"() -> (w1487:string[][])
                    n891 = property on="扭矩角度表格" class="Tbl (严格)"("Active Cell"=T2 {"Row"=4, "Column"=1} ("活动单元格:活动单元格"), "Cell BG Color"=u32 16711680 ("活动单元格:单元格背景色"), "Value"=w1487) -> ()  [unwired: 2 in, 2 out]
                  }
                }
              }
            }
            n892 = case shown="True" w1273 {
              frame False {
              }
              frame True {
                n893 = for {
                  N: 2 -> [_]
                  tunnel: [w1399] -> w1382
                  tunnel: [w1397] -> w1380
                  tunnel: [w1396] -> w1379
                  w1421 = 5 ("禁用的索引 (列)")
                  n894 = local read "扭矩字符串"() -> (w1420:string)
                  n895 = local read "角度字符串"() -> (w1419:string)
                  n896 = local read "扭矩/角度"() -> (w1425:string[][])
                  n897 = local read "已选产品"() -> (w1410:string[][])
                  n898 = Wait (ms)(milliseconds to wait=u32 1000 ("等待时间（毫秒）")) -> ()  [unwired: 1 out]
                  n899 = Fract/Exp String To Number(string=w1420) -> (number=w1405:dbl)  [unwired: 3 in, 1 out]
                  n900 = Fract/Exp String To Number(string=w1419) -> (number=w1400:dbl)  [unwired: 3 in, 1 out]
                  n901 = Index Array(array=w1410, index (row)=0 ("索引 (行)"), index (col)=4 ("禁用的索引 (列)")) -> (element=w1408:string)
                  n902 = Index Array(array=w1410, index (row)=0 ("索引 (行)"), index (col)=3 ("禁用的索引 (列)")) -> (element=w1409:string)
                  n903 = Index Array(array=w1410, index (row)=0 ("索引 (行)"), index (col)=6 ("禁用的索引 (列)")) -> (element=w1404:string)
                  n904 = Index Array(array=w1410, index (row)=0 ("索引 (行)"), index (col)=5 ("禁用的索引 (列)")) -> (element=w1403:string)
                  n905 = Fract/Exp String To Number(string=w1408) -> (number=w1407:dbl)  [unwired: 3 in, 1 out]
                  n906 = Fract/Exp String To Number(string=w1409) -> (number=w1406:dbl)  [unwired: 3 in, 1 out]
                  n907 = Fract/Exp String To Number(string=w1404) -> (number=w1402:dbl)  [unwired: 3 in, 1 out]
                  n908 = Fract/Exp String To Number(string=w1403) -> (number=w1401:dbl)  [unwired: 3 in, 1 out]
                  n909 = Replace Array Subset(array=w1425, new element #1=w1420, index (row) #1=w1421, index (col) #1=0 ("禁用的索引 (列)"), new element #2=w1419, index (row) #2=w1421, index (col) #2=1 ("索引 (列)")) -> (w1424:string[][])
                  n910 = In Range and Coerce(upper limit=w1407, x=w1405, lower limit=w1406) -> (In Range?=w1396:bool)  [unwired: 1 out]
                  n911 = In Range and Coerce(upper limit=w1402, x=w1400, lower limit=w1401) -> (In Range?=w1397:bool)  [unwired: 1 out]
                  n912 = local write "扭矩/角度"(w1424) -> ()
                  n913 = And(x=w1396, y=w1397) -> (x .and. y?=w1399:bool)
                }
                n914 = Not(x=w1382) -> (.not. x?=→"螺栓5读取错误":bool)
                n915 = case shown="False" w1382 {
                  tunnel: w1382 -> [_ w1428]
                  frame False {
                    n916 = property on="扭矩6合格" class="Bool (严格)"("Colors [4]"=cluster{u32, u32}[] [{16711680, 16711680}] ("颜色[4]")) -> ()  [unwired: 2 in, 2 out]
                  }
                  frame True {
                    n917 = local write "扭矩6合格"(w1428) -> ()
                    n918 = property on="扭矩6合格" class="Bool (严格)"("Colors [4]"=cluster{u32, u32}[] [{6618880, 6618880}] ("颜色[4]")) -> ()  [unwired: 2 in, 2 out]
                  }
                }
                n919 = case shown="False" w1379 {
                  frame True {
                    n920 = local read "扭矩/角度"() -> (w1390:string[][])
                    n921 = property on="扭矩角度表格" class="Tbl (严格)"("Active Cell"=T2 {"Row"=5, "Column"=0} ("活动单元格:活动单元格"), "Cell BG Color"=u32 6618880 ("活动单元格:单元格背景色"), "Value"=w1390) -> ()  [unwired: 2 in, 2 out]
                  }
                  frame False {
                    n922 = local read "扭矩/角度"() -> (w1393:string[][])
                    n923 = property on="扭矩角度表格" class="Tbl (严格)"("Active Cell"=T2 {"Row"=5, "Column"=0} ("活动单元格:活动单元格"), "Cell BG Color"=u32 16711680 ("活动单元格:单元格背景色"), "Value"=w1393) -> ()  [unwired: 2 in, 2 out]
                  }
                }
                n924 = case shown="False" w1380 {
                  frame True {
                    n925 = local read "扭矩/角度"() -> (w1384:string[][])
                    n926 = property on="扭矩角度表格" class="Tbl (严格)"("Active Cell"=T2 {"Row"=5, "Column"=1} ("活动单元格:活动单元格"), "Cell BG Color"=u32 6618880 ("活动单元格:单元格背景色"), "Value"=w1384) -> ()  [unwired: 2 in, 2 out]
                  }
                  frame False {
                    n927 = local read "扭矩/角度"() -> (w1387:string[][])
                    n928 = property on="扭矩角度表格" class="Tbl (严格)"("Active Cell"=T2 {"Row"=5, "Column"=1} ("活动单元格:活动单元格"), "Cell BG Color"=u32 16711680 ("活动单元格:单元格背景色"), "Value"=w1387) -> ()  [unwired: 2 in, 2 out]
                  }
                }
              }
            }
          }
          frame #1 {
            n929 = local read "已选产品"() -> (w1637:string[][])
            n930 = Index Array(array=w1637, index (row)=0 ("禁用的索引 (行)"), index (col)=7 ("禁用的索引 (列)")) -> (element=w1636:string)
            n931 = Decimal String To Number(string=w1636) -> (number=w1631:i32)  [unwired: 2 in, 1 out]
            n932 = Decrement(x=w1631) -> (x-1=w1630:i32)
            n933 = local read "扭矩/角度"() -> (w1635:string[][])
            n934 = Index Array(array=w1635, index (row)=w1630, index (col)=1 ("禁用的索引 (列)")) -> (element=w1633:string)
            n935 = String Length(string=w1633) -> (length=w1632:i32)
            n936 = Greater Than 0?(x=w1632) -> (x > 0?=w1629:bool)
            n937 = case shown="True" w1629 {
              frame False {
              }
              frame True {
                n938 = local read "已选产品"() -> (w1656:string[][])
                n939 = Index Array(array=w1656, index (row)=0 ("禁用的索引 (行)"), index (col)=7 ("禁用的索引 (列)")) -> (element=w1655:string)
                n940 = Decimal String To Number(string=w1655) -> (number=w1652:i32)  [unwired: 2 in, 1 out]
                n941 = case shown="7" w1652 {
                  tunnel: [_ w1709 w1717 w1724] -> w1658
                  frame 0, Default {
                  }
                  frame 6 {
                    n942 = local read "扭矩1合格"() -> (w1715:bool)
                    n943 = local read "扭矩2合格"() -> (w1714:bool)
                    n944 = local read "扭矩3合格"() -> (w1713:bool)
                    n945 = local read "扭矩4合格"() -> (w1712:bool)
                    n946 = local read "扭矩5合格"() -> (w1711:bool)
                    n947 = local read "扭矩6合格"() -> (w1710:bool)
                    n948 = Compound Arithmetic op=AND ("复合运算")(w1715, w1714, w1713, w1712, w1711, w1710) -> (w1709:bool)
                  }
                  frame 7 {
                    n949 = local read "扭矩1合格"() -> (w1723:bool)
                    n950 = local read "扭矩2合格"() -> (w1722:bool)
                    n951 = local read "扭矩3合格"() -> (w1721:bool)
                    n952 = local read "扭矩4合格"() -> (w1720:bool)
                    n953 = local read "扭矩5合格"() -> (w1719:bool)
                    n954 = local read "扭矩6合格"() -> (w1718:bool)
                    n955 = local read "扭矩7合格"() -> (w1716:bool)
                    n956 = Compound Arithmetic op=AND ("复合运算")(w1723, w1722, w1721, w1720, w1719, w1718, w1716) -> (w1717:bool)
                  }
                  frame 5 {
                    n957 = local read "扭矩1合格"() -> (w1729:bool)
                    n958 = local read "扭矩2合格"() -> (w1728:bool)
                    n959 = local read "扭矩3合格"() -> (w1727:bool)
                    n960 = local read "扭矩4合格"() -> (w1726:bool)
                    n961 = local read "扭矩5合格"() -> (w1725:bool)
                    n962 = Compound Arithmetic op=AND ("复合运算")(w1729, w1728, w1727, w1726, w1725) -> (w1724:bool)
                  }
                }
                n963 = call "数据查询.vi"() -> ("今日总数"=w1707:i32)  [unwired: 9 in, 2 out]
                n964 = Increment(x=w1707) -> (x+1=w1706:i32)
                n965 = Number To Decimal String(number=w1706, width (-)=i16 4 ("宽度(-)")) -> (decimal integer string=w1651:string)
                n966 = call <vilib>:"Space Constant.vi"() -> ("String"=w1650:string)
                n967 = case shown="True" w1658 {
                  tunnel: ["NG" "OK"] -> w1657
                  frame False {
                  }
                  frame True {
                  }
                }
                n968 = local read "扭矩/角度"() -> (w1642:string[][])
                n969 = local read "已选产品"() -> (w1664:string[][])
                n970 = Search and Replace String(replace all?=TRUE ("替换全部？(F)"), input string=w1651, search string=w1650, replace string="0") -> (result string=w1648:string)  [unwired: 4 in, 3 out]
                n971 = Format Date/Time String(time format string (%c)="%Y%m%d" ("时间格式字符串(%c)")) -> (date/time string=w1702:string)  [unwired: 2 in]
                n972 = property on="作业员 Operator" class="Ring (严格)"() -> ("RingText.Text"=w1660:string)  [unwired: 2 in, 2 out]
                n973 = Concatenate Strings(w1702, w1648) -> (w1701:string)
                n974 = Format Date/Time String(time format string (%c)="%Y%m%d %H:%M:%S" ("时间格式字符串(%c)")) -> (date/time string=w1704:string)  [unwired: 2 in]
                n975 = Index Array(array=w1642, index (row)=0 ("索引 (行)"), index (col)=0 ("禁用的索引 (列)")) -> (element=w1676:string)
                n976 = Index Array(array=w1642, index (row)=0 ("索引 (行)"), index (col)=1 ("禁用的索引 (列)")) -> (element=w1675:string)
                n977 = Index Array(array=w1642, index (row)=1 ("索引 (行)"), index (col)=0 ("禁用的索引 (列)")) -> (element=w1674:string)
                n978 = Index Array(array=w1642, index (row)=2 ("索引 (行)"), index (col)=0 ("禁用的索引 (列)")) -> (element=w1673:string)
                n979 = Index Array(array=w1642, index (row)=6 ("索引 (行)"), index (col)=1 ("禁用的索引 (列)")) -> (element=w1641:string)
                n980 = Index Array(array=w1642, index (row)=3 ("索引 (行)"), index (col)=0 ("禁用的索引 (列)")) -> (element=w1672:string)
                n981 = Index Array(array=w1642, index (row)=4 ("索引 (行)"), index (col)=0 ("禁用的索引 (列)")) -> (element=w1670:string)
                n982 = Index Array(array=w1664, index (row)=0 ("禁用的索引 (行)"), index (col)=0 ("禁用的索引 (列)")) -> (element=w1661:string)
                n983 = Index Array(array=w1642, index (row)=5 ("索引 (行)"), index (col)=1 ("禁用的索引 (列)")) -> (element=w1671:string)
                n984 = Index Array(array=w1642, index (row)=5 ("索引 (行)"), index (col)=0 ("禁用的索引 (列)")) -> (element=w1669:string)
                n985 = Index Array(array=w1642, index (row)=4 ("索引 (行)"), index (col)=1 ("禁用的索引 (列)")) -> (element=w1668:string)
                n986 = Index Array(array=w1642, index (row)=3 ("索引 (行)"), index (col)=1 ("禁用的索引 (列)")) -> (element=w1667:string)
                n987 = Index Array(array=w1642, index (row)=2 ("索引 (行)"), index (col)=1 ("禁用的索引 (列)")) -> (element=w1666:string)
                n988 = Index Array(array=w1642, index (row)=6 ("索引 (行)"), index (col)=0 ("禁用的索引 (列)")) -> (element=w1640:string)
                n989 = Index Array(array=w1642, index (row)=1 ("索引 (行)"), index (col)=1 ("禁用的索引 (列)")) -> (element=w1665:string)
                n990 = local read "二维码"() -> (w1659:string)
                n991 = call "数据库保存子vi.vi"("时间"=w1704, "序列号"=w1701, "二维码"=w1659, "扭矩1"=w1676, "角度1"=w1675, "扭矩2"=w1674, "角度2"=w1665, "扭矩3"=w1673, "扭矩7"=w1640, "角度7"=w1641, "角度3"=w1666, "扭矩4"=w1672, "角度4"=w1667, "扭矩5"=w1670, "角度5"=w1668, "扭矩6"=w1669, "人员"=w1660, "角度6"=w1671, "结果"=w1657, "产品型号"=w1661) -> ()
              }
            }
          }
          frame #2 {
            n992 = Wait (ms)(milliseconds to wait=u32 1000 ("等待时间（毫秒）")) -> ()  [unwired: 1 out]
          }
          frame #3 {
            n993 = case shown="True" w1734 {
              frame False {
              }
              frame True {
                w1735 = 0
                n994 = call "数据查询.vi"() -> ("今日合格数"=w1739:i32, "今日总数"=w1740:i32, "Data"=w1741:string[][])  [unwired: 9 in]
                n995 = local write "二维码长度"(w1735) -> ()
                n996 = local write "二维码"("") -> ()
                n997 = local write "表格"(w1741) -> ()
                n998 = local write "二维码对应程序号"(w1735) -> ()
                n999 = Number To Decimal String(number=w1740) -> (decimal integer string=w1738:string)  [unwired: 1 in]
                n1000 = Number To Decimal String(number=w1739) -> (decimal integer string=w1737:string)  [unwired: 1 in]
                n1001 = local write "今日总数"(w1738) -> ()
                n1002 = local write "今日合格"(w1737) -> ()
              }
            }
          }
          frame #4 {
            n1003 = local write "扭矩保存过程"(u8 2 ("扭矩保存过程")) -> ()
          }
        }
      }
    }
  }
  n1004 = call "IMAQ Dispose"("Image"=w4, "error in (no error)"=w5) -> ("error out"=→"error out 6":errorcluster)  [unwired: 4 in]
  n1005 = call "IMAQ Dispose"("Image"=w2, "error in (no error)"=w1) -> ("error out"=→"error out 4":errorcluster)  [unwired: 4 in]
